vi "PH_DataViewer.panel.vi"(0 "object ref":refnum<vi>, 5 "error in (no error)":errorcluster) -> (19 "error out":errorcluster)   [LabVIEW 2014, in "PH_DataViewer.lvlib"]
doc: "By this VI a hardware switch can be monitored and switched. \n\nThe indicators \"FALSE\", \"TRUE\" and \"SWITCH STATE\" show the value of the Beckhoff-Tag: blue indicates bad tag status reference problems, darkgreen false and lightgreen true. If everything is working fine, \"FALSE\" and \"SWITCH STATE\" should show the same value, while \"TRUE\" has the opposite value. The caption of the sensors for \"FALSE\" and \"TRUE\" are taken out of the database. In case of only one or no sensor these GUI elements are not shown at all.\n\nThe oval button switches. It should be in the same state as the \"SWITCH STATE\" indicator. \n\n\"Delete Instance\" disconnects and removes the instance from the PCS.\n\n\nLicense Agreement for this software:\n\nCopyright (C)\nGesellschaft für Schwerionenforschung, GSI\nPlanckstr. 1\n64291 Darmstadt\nGermany\n\nContact: D.Beck@gsi.de \n\nThis program is free software; you can redistribute it and/or modify it under the terms of the GNU General Public License as published by the Free Software Foundation; either version 2 of the license, or (at your option) any later version.\n\nThis program is distributed in the hope that it will be useful, but WITHOUT ANYW ARRANTY; without even the implied warranty of MERCHANTABILITY or FITNESS FOR A PARTICULAR PURPOSE. See the GNU General License for more details (http://www.gnu.org).\n\nGesellschaft für Schwerionenforschung, GSI\nPlanckstr. 1, 64291 Darmstadt, Germany\nFor all questions and ideas contact: M.Richter@gsi.de, H.Brand@gsi.de or D.Beck@gsi.de.\nLast update: 18-DEC-2002"
uses:
  PH_DataViewer.lvlib
  PH_Calorimeter_USB/PH_Calorimeter_USB.Channel.ctl
  PH_Calorimeter_USB/PH_Calorimeter_USB.Channel Gain.ctl
  PH_gentec_Powermeter.Data.ctl
  PH_DataViewer.Device State.ctl
  PH_Common.PP PU Data.ctl
  PH_Basics/PH_StatusHandler/PH_StatusHandler.Status.ctl
  PH_PP_Trigger.Data.ctl
  PH_VacuumControl.Data.ctl
  PH_Blackbox.Data.ctl
  PH_PA_Chiller.Data.ctl
  PH_IEEE1394Camera.Data.ctl
  PH_IEEE1394Camera.Settings.ctl
  PH_ImageOperator.Data.ctl
  PH_Vision/PH_ImageCalibrator/PH_ImageCalibrator.Calibration Data - Version 1.ctl
  PH_Vision/PH_ImageOperator/PH_ImageOperator.Beam Analysis Data.ctl
  BNC555.Data.ctl
  PH_Common.PP PU Data Vers2.ctl
  PH_Sequencer.Data.ctl
  PH_BackreflectionMeas.Data.ctl
  PH_OceanOpticsSpectrometer.Data.ctl
  CS_Core/CSObj/CSObj.lvlib
  PH_Basics/PH_Common/PH_Common.lvlib
  PHELIX/PH_BackreflectionMeas/PH_BackreflectionMeas.lvlib
  PH_Devices/PH_OceanOpticsSpectrometer/PH_OceanOpticsSpectrometer.lvlib
  PH_Calorimeter_USB/PH_Calorimeter_USB.lvlib
  PH_Vision/PH_ImageOperator/PH_ImageOperator.lvlib
  PH_Basics/PH_StatusHandler/PH_StatusHandler.lvlib
  PH_Vision/PH_ImageCalibrator/PH_ImageCalibrator.lvlib
panel:
  out "OO Spectrometer":T1[](array[typedef])
  out "Backreflection Meas":T2[](array[typedef]) {"Waveform Data"."Initial X" format="%.2e"}
  in  "PP PU Data Version 2":T3={"Instance"="N/A", "Snapshot: Date"="N/A", "Snapshot: Time"="N/A", "PU in use?"=FALSE, "Time betweeen Shots [Min]"=0.0, "Waiting Time over?"=FALSE, "Voltage [V]"=0.0, "State"=0, "Timeout SM"=""} {"State" items=["no info", "off/false/out", "on/true/in", "Failure", "Alarm", "Status 1", "Status 2", "Status 3"]}
  out "f 2":dbl caption="mm"
  out "M":dbl
  out "Img Operators":T5[](array[typedef]) {"Energy"."State" items=["no info", "off/false", "on/true", "Failure", "Alarm"]; "Cam Settings"."Serial Number" format="%#_12g"; "Calibration"."Calibration data - Version 1"."Cam Settings"."Serial Number" format="%#_12g"; "Calibration"."Status" items=["no info", "off/false", "on/true", "Failure", "Alarm"]}
  out "Cams":T9[](array[typedef]) {"Cam Settings"."Serial Number" format="%#_12g"}
  out "PP PUs":T11[](array[typedef]) {"State" items=["no info", "off/false/out", "on/true/in", "Failure", "Alarm", "Status 1", "Status 2", "Status 3"]}
  out "Powermeters":T12[](array[typedef]) {"Device State" items=["no info", "off/false", "on/true", "Failure", "Alarm"]}
  in  "Empty":waveform(dbl)[](array[waveform])
  out "Current Meas Data":waveform(dbl)[][](array[waveform])
  in  "Main Tab":T13(tab)
  out "Sequencer Data":T14={"Instance"="N/A", "Snapshot: Date"="N/A", "Snapshot: Time"="N/A", "Shot Comment"=""}
  in  "Tab Opt Diagn":T15(tab)
  out "Time Calo":string
  out "Date Calo":string
  out "Graph":cluster{"Raw Data":dbl[], "Raw Data":dbl[]}(graph)
  out "Energy [J]":dbl format="%.3f"
  out "PH Calorimeter Device Config":T18 {"Channel Gain" items=["Range: +/- 10 V", "Range: +/- 2.5 V ", "Range: +/- 1 V", "Range: +/- 0.25 V", "Range: +/- 0.1 V", "Range: +/- 0.025 V"]; "Channel" items=["Channel 1", "Channel 2", "Channel 3", "Channel 4", "Channel 5", "Channel 6", "Channel 7", "Channel 8", "Channel 9", "Channel 10", "Channel 11", "Channel 12", "Channel 13", "Channel 14", "Channel 15", "Channel 16"]}
  out "Status Powermeter":u32(colorbox) caption="Powermeter"
  in  "Powermeter":u16(ring)
  out "Unit":string
  out "Current Value":dbl format="%#_3f"
  out "Serial Number":string
  out "Scaling Factor":dbl format="%#.3f"
  out "Trigger Level":dbl format="%#.3f"
  out "Time Powermeter":string
  out "Date Powermeter":string
  in  "Export Img Data":bool caption="Export Data"
  out "Cam Trigger":T19 caption="Trigger"
  out "Cam Settings":T20 caption="Settings" {"Serial Number" format="%#_15g"}
  in  "Cameras":u16(ring)
  out "Time Cams":string
  out "Date Cams":string
  out "Cam Image":T21(plugin-control) caption="Image"
  in  "Tab Img Op":T22(tab)
  in  "Export Op Img":bool caption="Export Data"
  out "Bg subtracted":bool
  out "Op Image":T21(plugin-control) caption="Image"
  out "f rel to major?":bool
  out "Energy":dbl caption="PiS" format="%#_8g"
  out "exp Energy":dbl caption="mJ"
  out "Energy on":bool caption="Energy"
  out "Analysis Type":u16(ring) items=["over all", "ROI"]
  out "BA: Factor for ROI":i32=3 caption="Factor"
  out "BA: Steps":i32=3 caption="Steps"
  out "CoG - Y":dbl caption="Pix"
  out "CoG - X":dbl caption="Pix"
  out "e":dbl caption="PixSum"
  out "f":dbl caption="°"
  out "Min Diam":dbl caption="Pix"
  out "Maj Diam":dbl caption="Pix"
  out "Beam Analysis":bool caption="Analysis"
  out "Position Type":u16(ring) items=["Nearfield", "Farfield"]
  out "D":dbl caption="mm"
  out "q":dbl caption="mrad"
  out "exp - Y":i32 caption="Pix"
  out "exp - X":i32 caption="Pix"
  out "Position":bool
  out "Min 1 %":dbl caption="Pix"
  out "Maj 1 %":dbl caption="Pix"
  out "Fit Gauss":bool
  out "Min Fit Order":i32
  out "Maj Fit Order":i32
  out "Min FWHM":dbl caption="Pix"
  out "Maj FWHM":dbl caption="Pix"
  in  "Export Min Trace":bool caption="Export Min"
  in  "Export Maj Trace":bool caption="Export Maj"
  out "Minor Trace":cluster{"Index":sgl[], dbl[]}[](graph)
  out "Major Trace":cluster{"Index":sgl[], dbl[]}[](graph)
  out "Cam Settings Operator":T20 caption="Settings" {"Serial Number" format="%#_15g"}
  out "Background Image":T21(plugin-control) caption="Image"
  in  "Export BG Img":bool caption="Export BG Image"
  out "Status Cali Data":T6 caption="Status" items=["no info", "off/false", "on/true", "Failure", "Alarm"]
  out "Calibration data":T23 {"Cam Settings"."Serial Number" format="%#_12g"}
  in  "Operators":u16(ring)
  out "Time Operators":string
  out "Date Operators":string
  in  "Export Data BRM":bool caption="Export Data"
  out "BRM Graph":waveform(dbl)[](graph)
  in  "Backreflection Measurement":u16(ring)
  out "Time BRM":string
  out "Date BRM":string
  in  "OO Spectrometer Instancelist":u16(ring)
  out "Time OO Spectro":string
  out "Date OO Spectro":string
  in  "Export OO Spectro Data":bool caption="Export Data"
  out "OO Spectrum":cluster{"Wavelength Bins":sgl[], sgl[]}(graph)
  in  "Tab PP":enum32{"Current Meas", "Power Units", "Misc"}(tab)
  in  "Export Current Meas Data":bool caption="Export Data"
  in  "Power Unit CM":u16(ring)
  out "current meas data indicator":waveform(dbl)[](graph) caption="Measurement data"
  out "Time Current Meas":string
  out "Date Current Meas":string
  out "Waiting Time [Min]":dbl
  out "State after Shot":T4 caption="PPMA Sequencer State" items=["no info", "off/false/out", "on/true/in", "Failure", "Alarm", "Status 1", "Status 2", "Status 3"]
  out "Timeout SM":string
  out "in use after Shot":bool caption="still on?"
  out "Time PU after Shot":string
  out "Date PU after Shot":string
  out "State before Shot":T4 caption="PPMA Sequencer State" items=["no info", "off/false/out", "on/true/in", "Failure", "Alarm", "Status 1", "Status 2", "Status 3"]
  out "Delay [s]":dbl
  out "Voltage [V]":dbl
  out "Waiting Time over":bool
  out "in use before Shot":bool caption="in use"
  out "Time PU before Shot":string
  out "Date PU before Shot":string
  out "Gate Gen Chan":string
  in  "Power Unit":u16(ring)
  out "Mercury Monitor":T24={"Device"="N/A", "Snapshot: Date"="N/A", "Snapshot: Time"="N/A", "State On/Off"=0, "State Alarm"=0, "Concentration [mg/m³]"=0.0, "On since"="N/A"} {"Concentration [mg/m³]" format="%#_9g"; "State Alarm" items=["no info", "off/false", "on/true", "Failure", "Alarm"]; "State On/Off" items=["no info", "off/false", "on/true", "Failure", "Alarm"]}
  out "Triggers":T25[](array[typedef])
  in  "Tab Timing":enum32{"BNC 555s", "SRDG 535s"}(tab)
  out "BNC555s":T27(array[cluster]) {"BNC555 ConfigData"."Configuration"."System"."To Gate Polarity" items=["Low", "High"]; "BNC555 ConfigData"."Configuration"."System"."To Trigger Edge" items=["Rising", "Falling"]; "BNC555 ConfigData"."Configuration"."System"."To Trigger Threshold" min=0.2 max=12 step=0.01 format="%.2f"; "BNC555 ConfigData"."Configuration"."System"."To DCycle Off Count" min=1 max=50000 step=1; "BNC555 ConfigData"."Configuration"."System"."To DCycle On Count" min=1 max=50000 step=1; "BNC555 ConfigData"."Configuration"."System"."To Burst Count" min=1 max=50000 step=1; "BNC555 ConfigData"."Configuration"."System"."To Trigger Mode" items=["Disabled", "Trigger", "Gate"]; "BNC555 ConfigData"."Configuration"."System"."To Mode" items=["Normal", "Single", "Burst", "DCycle"]; "BNC555 ConfigData"."Configuration"."System"."To Period" min=1e-06 max=20.0 step=1e-07 format="%.7f"; "BNC555 ConfigData"."Configuration"."System"."To State" items=["Disabled", "Enable"]; "BNC555 ConfigData"."Channel Array"."Channel Setup"."Ch Divide By Count" min=1 max=50000 step=1; "BNC555 ConfigData"."Channel Array"."Channel Setup"."Ch Burst Count" min=1 max=50000 step=1; "BNC555 ConfigData"."Channel Array"."Channel Setup"."Ch Mode" items=["Normal", "Single", "Burst", "Divide by"]; "BNC555 ConfigData"."Channel Array"."Channel Setup"."Ch Gate" items=["Disabled", "Enabled"]; "BNC555 ConfigData"."Channel Array"."Channel Setup"."Ch Gate Polarity" items=["Normal", "Complement"]; "BNC555 ConfigData"."Channel Array"."Channel Setup"."Ch Polarity" items=["Normal", "Complement"]; "BNC555 ConfigData"."Channel Array"."Channel Setup"."Ch Amplitude" min=1.99 max=12 step=0.01 format="%.2f"; "BNC555 ConfigData"."Channel Array"."Channel Setup"."Ch Output" items=["TTL", "Adjustable"]; "BNC555 ConfigData"."Channel Array"."Channel Setup"."Ch Delay" min=0.0 max=20.0 step=1e-09 format="%.9f"; "BNC555 ConfigData"."Channel Array"."Channel Setup"."Ch Width" min=4e-09 max=20.0 step=1e-09 format="%.9f"; "BNC555 ConfigData"."Channel Array"."Channel Setup"."Ch State" items=["Disabled", "Enable"]}
  out "SRDGs":T28(array[cluster]) {"Trigger Settings"."Burst Period" min=4 max=32766; "Trigger Settings"."Internal/Burst Rate (Hz)" min=0.001 max=1000000.0 format="%.3f"; "Trigger Settings"."external level (V)" min=-2.56 max=2.56 format="%.2f"; "Trigger Settings"."burst count" min=2 max=32766; "Trigger Settings"."trigger" scale=0.0..4.0; "Output Settings"."CH CD"."Mode" items=["TTL", "NIM", "ECL", "VAR"]; "Output Settings"."CH CD"."Offset (V)" min=-3.0 max=4.0 format="%.2f"; "Output Settings"."CH CD"."Amplitude (V)" min=-3.0 max=4.0 format="%.2f"; "Output Settings"."CH D"."Mode" items=["TTL", "NIM", "ECL", "VAR"]; "Output Settings"."CH D"."Offset (V)" min=-3.0 max=4.0 format="%.2f"; "Output Settings"."CH D"."Amplitude (V)" min=-3.0 max=4.0 format="%.2f"; "Output Settings"."CH C"."Mode" items=["TTL", "NIM", "ECL", "VAR"]; "Output Settings"."CH C"."Offset (V)" min=-3.0 max=4.0 format="%.2f"; "Output Settings"."CH C"."Amplitude (V)" min=-3.0 max=4.0 format="%.2f"; "Output Settings"."CH AB"."Mode" items=["TTL", "NIM", "ECL", "VAR"]; "Output Settings"."CH AB"."Offset (V)" min=-3.0 max=4.0 format="%.2f"; "Output Settings"."CH AB"."Amplitude (V)" min=-3.0 max=4.0 format="%.2f"; "Output Settings"."CH B"."Mode" items=["TTL", "NIM", "ECL", "VAR"]; "Output Settings"."CH B"."Offset (V)" min=-3.0 max=4.0 format="%.2f"; "Output Settings"."CH B"."Amplitude (V)" min=-3.0 max=4.0 format="%.2f"; "Output Settings"."CH A"."Mode" items=["TTL", "NIM", "ECL", "VAR"]; "Output Settings"."CH A"."Offset (V)" min=-3.0 max=4.0 format="%.2f"; "Output Settings"."CH A"."Amplitude (V)" min=-3.0 max=4.0 format="%.2f"; "Output Settings"."CH T0"."Mode" items=["TTL", "NIM", "ECL", "VAR"]; "Output Settings"."CH T0"."Offset (V)" min=-3.0 max=4.0 format="%.2f"; "Output Settings"."CH T0"."Amplitude (V)" min=-3.0 max=4.0 format="%.2f"; "Delay Settings"."CH D"."Delay (s)" format="%#_13g"; "Delay Settings"."CH D"."rel to" scale=0.0..3.0; "Delay Settings"."CH C"."Delay (s)" format="%#_13g"; "Delay Settings"."CH C"."rel to" scale=0.0..3.0; "Delay Settings"."CH B"."Delay (s)" format="%#_13g"; "Delay Settings"."CH B"."rel to" scale=0.0..3.0; "Delay Settings"."CH A"."Delay (s)" format="%#_13g"; "Delay Settings"."CH A"."rel to" scale=0.0..3.0}
  out "Chillers":T29[](array[typedef]) {"State Niveau" items=["no info", "off/false", "on/true", "Failure", "Alarm"]; "State Temperature" items=["no info", "off/false", "on/true", "Failure", "Alarm"]; "State Conductivity" items=["no info", "off/false", "on/true", "Failure", "Alarm"]; "State Flow" items=["no info", "off/false", "on/true", "Failure", "Alarm"]}
  out "Vac Controls":T30[](array[typedef])
  out "Black Boxes":T31[](array[typedef]) {"Status" items=["no info", "off/false", "on/true", "Failure", "Alarm", "Status 1", "Status 2", "Status 3"]}
  out "Path/File":path
  in  "Read Data":bool
  in  "Delete":bool
  out "loop counter":i32
  # "PCS"
  # "3.40"
  # "before Shot"
  # "after Shot"
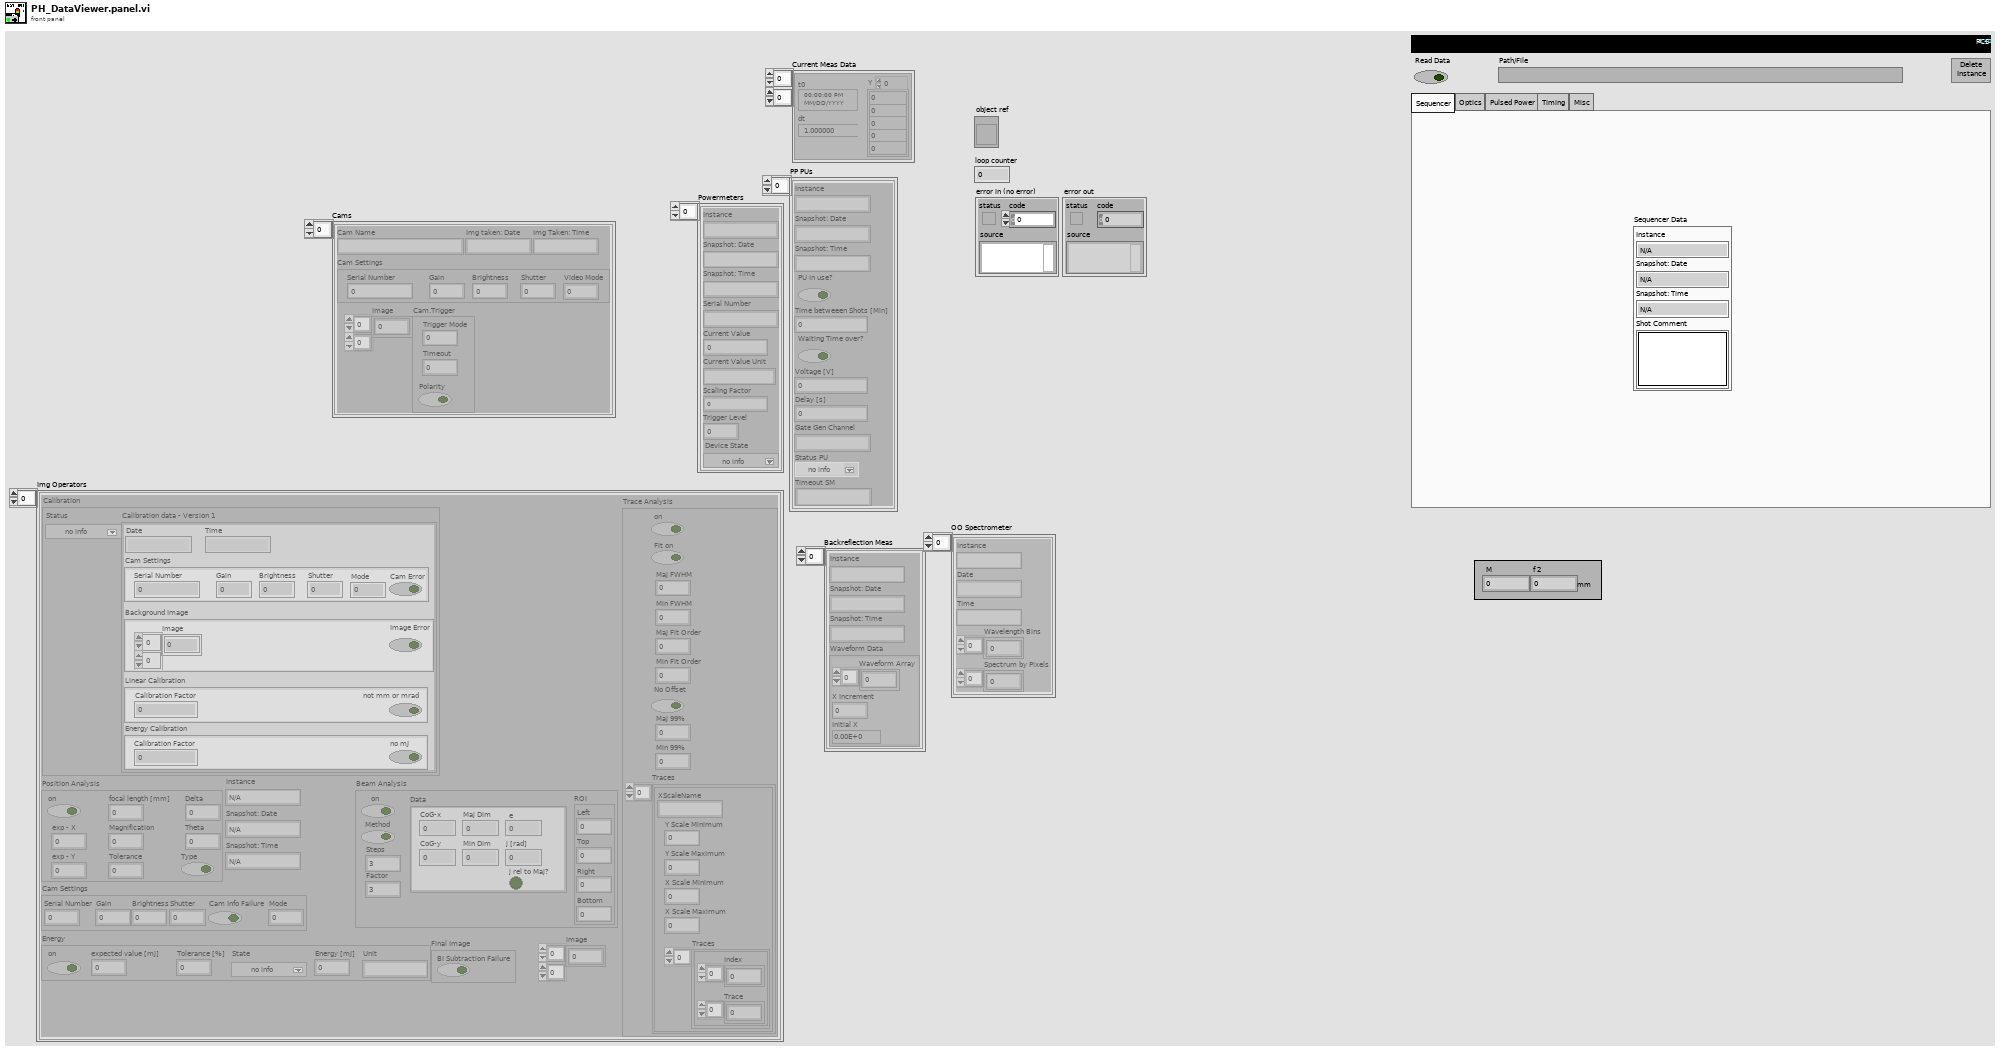
[diagram p1: front panel]
types:
  T1 = typedef "PH_DataViewer.lvlib/PH_OceanOpticsSpectrometer.Data.ctl" = cluster{"Instance":string, "Date":string, "Time":string, "Wavelength Bins":dbl[], "Spectrum by Pixels":dbl[]}
  T2 = typedef "PH_DataViewer.lvlib/PH_BackreflectionMeas.Data.ctl" = cluster{"Instance":string, "Snapshot: Date":string, "Snapshot: Time":string, "Waveform Data":cluster{"Waveform Array":dbl[], "X Increment":dbl, "Initial X":dbl}}
  T3 = typedef "PH_DataViewer.lvlib/PH_Common.PP PU Data Vers2.ctl" = cluster{"Instance":string, "Snapshot: Date":string, "Snapshot: Time":string, "PU in use?":bool, "Time betweeen Shots [Min]":dbl, "Waiting Time over?":bool, "Voltage [V]":dbl, "State":T4, "Timeout SM":string}
  T4 = typedef "PH_StatusHandler.lvlib/PH_StatusHandler.Status.ctl" = i16
  T5 = typedef "PH_DataViewer.lvlib/PH_ImageOperator.Data.ctl" = cluster{"Instance":string, "Snapshot: Date":string, "Snapshot: Time":string, "Calibration":cluster{"Status":T6, "Calibration data - Version 1":T7}, "Position Analysis":cluster{"on":bool, "exp - X":i32, "exp - Y":i32, "focal length [mm]":dbl, "Magnification":dbl, "Delta":dbl, "Theta":dbl, "Tolerance":dbl, "Type":bool}, "Beam Analysis":cluster{"on":bool, "Data":T8, "Method":bool, "Steps":i32, "Factor":i32, "ROI":cluster{"Left":i32, "Top":i32, "Right":i32, "Bottom":i32}}, "Cam Settings":cluster{"Serial Number":dbl, "Gain":i32, "Brightness":i32, "Shutter":i32, "Cam Info Failure":bool, "Mode":i32}, "Energy":cluster{"on":bool, "expected value [mJ]":dbl, "Tolerance [%]":dbl, "State":T6, "Energy [mJ]":dbl, "Unit":string}, "Image":dbl[][], "Final Image":cluster{"BI Subtraction Failure":bool}, "Trace Analysis":cluster{"on":bool, "Fit on":bool, "Maj FWHM":dbl, "Min FWHM":dbl, "Maj Fit Order":i32, "Min Fit Order":i32, "No Offset":bool, "Maj 99%":dbl, "Min 99%":dbl, "Traces":cluster{"XScaleName":string, "Y Scale Minimum":sgl, "Y Scale Maximum":sgl, "X Scale Minimum":sgl, "X Scale Maximum":sgl, "Traces":cluster{"Index":sgl[], "Trace":dbl[]}[]}[]}}
  T6 = typedef "PH_DataViewer.lvlib/PH_DataViewer.Device State.ctl" = i32
  T7 = typedef "PH_ImageCalibrator.lvlib/PH_ImageCalibrator.Calibration Data - Version 1.ctl" = cluster{"Date":string, "Time":string, "Cam Settings":cluster{"Serial Number":dbl, "Gain":i32, "Brightness":i32, "Shutter":i32, "Cam Error":bool, "Mode":i32}, "Background Image":cluster{"Image":dbl[][], "Image Error":bool}, "Linear Calibration":cluster{"Calibration Factor":dbl, "not mm or mrad":bool}, "Energy Calibration":cluster{"Calibration Factor":dbl, "no mJ":bool}}
  T8 = typedef "PH_ImageOperator.lvlib/PH_ImageOperator.Beam Analysis Data.ctl" = cluster{"CoG-x":sgl, "CoG-y":sgl, "Maj Dim":dbl, "Min Dim":dbl, "Ellipticity":dbl, "Azimuth Angle [rad]":dbl, "Azi Angle rel to Maj?":bool}
  T9 = typedef "PH_DataViewer.lvlib/PH_IEEE1394Camera.Data.ctl" = cluster{"Cam Name":string, "Img taken: Date":string, "Img Taken: Time":string, "Cam Settings":T10, "Image":sgl[][], "Cam.Trigger":cluster{"Trigger Mode":u16, "Timeout":u32, "Polarity":bool}}
  T10 = typedef "PH_DataViewer.lvlib/PH_IEEE1394Camera.Settings.ctl" = cluster{"Serial Number":dbl, "Gain":i32, "Brightness":i32, "Shutter":i32, "Video Mode":i32}
  T11 = typedef "PH_DataViewer.lvlib/PH_Common.PP PU Data.ctl" = cluster{"Instance":string, "Snapshot: Date":string, "Snapshot: Time":string, "PU in use?":bool, "Time betweeen Shots [Min]":dbl, "Waiting Time over?":bool, "Voltage [V]":dbl, "Delay [s]":dbl, "Gate Gen Channel":string, "State":T4, "Timeout SM":string}
  T12 = typedef "PH_DataViewer.lvlib/PH_gentec_Powermeter.Data.ctl" = cluster{"Instance":string, "Snapshot: Date":string, "Snapshot: Time":string, "Serial Number":string, "Current Value":dbl, "Current Value Unit":string, "Scaling Factor":dbl, "Trigger Level":dbl, "Device State":T6}
  T13 = enum32{"Sequencer", "Optics", "Pulsed Power", "Timing", "Misc"}
  T14 = typedef "PH_DataViewer.lvlib/PH_Sequencer.Data.ctl" = cluster{"Instance":string, "Snapshot: Date":string, "Snapshot: Time":string, "Shot Comment":string}
  T15 = enum32{"Calorimeter", "Powermeter", "Cams", "Operator", "Backreflection Meas", "OO Spectrometer"}
  T16 = typedef "PH_Calorimeter_USB.lvlib/PH_Calorimeter_USB.Channel.ctl" = u16
  T17 = typedef "PH_Calorimeter_USB.lvlib/PH_Calorimeter_USB.Channel Gain.ctl" = u16
  T18 = cluster{"Channel":T16, "Channel Gain":T17, "Device name":string, "Sensitivity [Vs/J]":dbl, "T 1/e [s]":dbl, "Serial No.":string}
  T19 = cluster{"Trigger Mode":u16, "Timeout":u32, "Polarity":bool}
  T20 = cluster{"Serial Number":dbl, "Gain":i32, "Brightness":i32, "Shutter":i32, "Mode":i32}
  T21 = typedef "IMAQ Image.ctl" = refnum<image>
  T22 = enum32{"Image", "Results", "Traces", "Cam Settings", "Bg Img", "Cali data"}
  T23 = cluster{"Date":string, "Time":string, "Cam Settings":cluster{"Serial Number":dbl, "Gain":i32, "Brightness":i32, "Shutter":i32, "Cam Error":bool, "Mode":i32}, "Background Image":cluster{"Image":dbl[][], "Image Error":bool}, "Linear Calibration":cluster{"Calibration Factor":dbl, "not mm nor mrad":bool}, "Energy Calibration":cluster{"Calibration Factor":dbl, "no mJ":bool}}
  T24 = cluster{"Device":string, "Snapshot: Date":string, "Snapshot: Time":string, "State On/Off":T6, "State Alarm":T6, "Concentration [mg/m³]":dbl, "On since":string}
  T25 = typedef "PH_DataViewer.lvlib/PH_PP_Trigger.Data.ctl" = cluster{"Instance":string, "Snapshot: Date":string, "Snapshot: Time":string, "last shot":string}
  T26 = typedef "PH_DataViewer.lvlib/BNC555.Data.ctl" = cluster{"Channel Array":cluster{"channel name (\"A\")":string, "Channel Setup":cluster{"Ch State":i8, "Ch Width":dbl, "Ch Delay":dbl, "Ch Output":i8, "Ch Amplitude":sgl, "Ch Polarity":i8, "Ch Gate Polarity":i8, "Ch Gate":i8, "Ch Mode":i8, "Ch Burst Count":i32, "Ch Divide By Count":i32}}[], "Configuration":cluster{"System":cluster{"To State":i8, "To Period":dbl, "To Mode":i8, "To Trigger Mode":i8, "To Burst Count":i32, "To DCycle On Count":i32, "To DCycle Off Count":i32, "To Trigger Threshold":sgl, "To Trigger Edge":i8, "To Gate Polarity":i8}}}
  T27 = cluster{"Object":string, "BNC555 ConfigData":T26}[]
  T28 = cluster{"Instance":string, "Snapshot: Date":string, "Snapshot: Time":string, "Delay Settings":cluster{"CH A":cluster{"rel to":u32, "Delay (s)":dbl}, "CH B":cluster{"rel to":u32, "Delay (s)":dbl}, "CH C":cluster{"rel to":u32, "Delay (s)":dbl}, "CH D":cluster{"rel to":u32, "Delay (s)":dbl}}, "Output Settings":cluster{"CH T0":cluster{"Inversion":bool, "Amplitude (V)":dbl, "Offset (V)":dbl, "Mode":i32, "Load":bool}, "CH A":cluster{"Inversion":bool, "Amplitude (V)":dbl, "Offset (V)":dbl, "Mode":i32, "Load":bool}, "CH B":cluster{"Inversion":bool, "Amplitude (V)":dbl, "Offset (V)":dbl, "Mode":i32, "Load":bool}, "CH AB":cluster{"Inversion":bool, "Amplitude (V)":dbl, "Offset (V)":dbl, "Mode":i32, "Load":bool}, "CH C":cluster{"Inversion":bool, "Amplitude (V)":dbl, "Offset (V)":dbl, "Mode":i32, "Load":bool}, "CH D":cluster{"Inversion":bool, "Amplitude (V)":dbl, "Offset (V)":dbl, "Mode":i32, "Load":bool}, "CH CD":cluster{"Inversion":bool, "Amplitude (V)":dbl, "Offset (V)":dbl, "Mode":i32, "Load":bool}}, "Trigger Settings":cluster{"trigger":u32, "Impedance":bool, "Slope":bool, "burst count":i32, "external level (V)":sgl, "Internal/Burst Rate (Hz)":dbl, "Burst Period":i32}}[]
  T29 = typedef "PH_DataViewer.lvlib/PH_PA_Chiller.Data.ctl" = cluster{"Instance":string, "Snapshot: Date":string, "Snapshot: Time":string, "State Flow":T6, "State Conductivity":T6, "State Temperature":T6, "State Niveau":T6}
  T30 = typedef "PH_DataViewer.lvlib/PH_VacuumControl.Data.ctl" = cluster{"Instance":string, "Snapshot: Date":string, "Snapshot: Time":string, "Channels":cluster{"Gauge":string, "Value (mbar)":dbl, "Limit (mbar)":dbl}[]}
  T31 = typedef "PH_DataViewer.lvlib/PH_Blackbox.Data.ctl" = cluster{"Instance":string, "Snapshot: Date":string, "Snapshot: Time":string, "Remote Controlled?":bool, "Status":i32}
  T32 = typedef "PH_DataViewer.lvlib/PH_DataViewer.i attribute.ctl" = cluster{"Images":cluster{"CAM":cluster{string, u32}, "BACKGROUND":cluster{string, u32}, "OPERATOR":cluster{string, u32}}, "Cam Operator GUI Refs":cluster{"Date Operators":refnum<vi>, "Time Operators":refnum<vi>, "Status Cali Data":refnum<vi>, "Calibration data":refnum<vi>, "Background Image":refnum<vi>, "Bg subtracted":refnum<vi>, "Op Image":refnum<vi>, "Cam Settings Operator":refnum<vi>, "Energy on":refnum<vi>, "exp Energy":refnum<vi>, "Energy":refnum<vi>, "Beam Analysis":refnum<vi>, "Analysis Type":refnum<vi>, "BA: Steps":refnum<vi>, "BA: Factor for ROI":refnum<vi>, "CoG - X":refnum<vi>, "CoG - Y":refnum<vi>, "Maj Diam":refnum<vi>, "Min Diam":refnum<vi>, "Phi":refnum<vi>, "Epsilon":refnum<vi>, "Phi rel to maj":refnum<vi>, "Position":refnum<vi>, "Position Type":refnum<vi>, "exp - X":refnum<vi>, "exp - Y":refnum<vi>, "Magni":refnum<vi>, "Foc Length":refnum<vi>, "Delta":refnum<vi>, "Theta":refnum<vi>, "Fit Gauss":refnum<vi>, "Maj Fit Order":refnum<vi>, "Min Fit Order":refnum<vi>, "Maj FWHM":refnum<vi>, "Min FWHM":refnum<vi>, "Maj 1 %":refnum<vi>, "Min 1 %":refnum<vi>}}
  T33 = typedef "PH_DataViewer.lvlib/PH_Calorimater_USB.Data.ctl" = cluster{"PH Calorimeter Device Config":T34, "Output Rate [Hz]":i32, "Offset time [s]":dbl, "Taken + Calc: Date":string, "Taken + Calc: Time":string, "Raw Data":dbl[][], "Energy [J]":dbl}
  T34 = typedef "PH_Calorimeter_USB.lvlib/PH_Calorimeter_USB.Device Config.ctl" = cluster{"Channel":T16, "Channel Gain":T17, "Device name":string, "Sensitivity":dbl, "T 1/e":dbl, "Serial No.":string}
  T35 = typedef "PH_DataViewer.lvlib/PH_CurrentMeas.Data.ctl" = cluster{"Instance":string, "Snapshot: Date":string, "Snapshot: Time":string, "PU Data":cluster{"Data":waveform(dbl)[], "PU Name":string}[]}
  T36 = typedef "PH_DataViewer.lvlib/PH_Mercury_Monitor.Data.ctl" = cluster{"Device":string, "Snapshot: Date":string, "Snapshot: Time":string, "State On/Off":T6, "State Alarm":T6, "Concentration [mg/m³]":dbl, "On since":string}
  T37 = cluster{"Black Boxes":T31[], "Calorimeters":T33[], "Current Meas'":T35[], "Powermeters":T12[], "Cams":T9[], "Img Operators":T5[], "Mercury Monitors":T36[], "Chillers":T29[], "Triggers":T25[], "Vac Controls":T30[], "PP PUs":T11[], "BNC555s":cluster{"Object":string, "BNC555 ConfigData":T26}[]}
  T38 = typedef "PH_DataViewer.lvlib/PHELIX_Data_Vers2.ctl" = cluster{"Black Boxes":T31[], "Calorimeters":T33[], "Current Meas'":T35[], "Powermeters":T12[], "Cams":T9[], "Img Operators":T5[], "Mercury Monitors":T36[], "Chillers":T29[], "Triggers":T25[], "Vac Controls":T30[], "PP PUs":T3[], "BNC555s":cluster{"Object":string, "BNC555 ConfigData":T26}[], "SRDG535s":T39[], "Sequencer Data":T14}
  T39 = typedef "PH_DataViewer.lvlib/SRDG535.Data.ctl" = cluster{"Instance":string, "Snapshot: Date":string, "Snapshot: Time":string, "Delay Settings":T40, "Output Settings":T41, "Trigger Settings":T43}
  T40 = typedef "SRDG535.lvlib/SRDG535.Delay.ctl" = cluster{"CH A":cluster{"rel to":u32, "Delay (s)":dbl}, "CH B":cluster{"rel to":u32, "Delay (s)":dbl}, "CH C":cluster{"rel to":u32, "Delay (s)":dbl}, "CH D":cluster{"rel to":u32, "Delay (s)":dbl}}
  T41 = typedef "SRDG535.lvlib/SRDG535.Output.ctl" = cluster{"CH T0":T42, "CH A":T42, "CH B":T42, "CH AB":T42, "CH C":T42, "CH D":T42, "CH CD":T42}
  T42 = typedef "SRDG535.lvlib/SRDG535.Channel Output.ctl" = cluster{"Inversion":bool, "Amplitude (V)":dbl, "Offset (V)":dbl, "Mode":i32, "Load":bool}
  T43 = typedef "SRDG535.lvlib/SRDG535.Trigger.ctl" = cluster{"trigger":u32, "Impedance":bool, "Slope":bool, "burst count":i32, "external level (V)":sgl, "Internal/Burst Rate (Hz)":dbl, "Burst Period":i32}
  T44 = typedef "PH_DataViewer.lvlib/PHELIX_Data_Vers3.ctl" = cluster{"Black Boxes":T31[], "Calorimeters":T33[], "Current Meas'":T35[], "Powermeters":T12[], "Cams":T9[], "Img Operators":T5[], "Mercury Monitors":T36[], "Chillers":T29[], "Triggers":T25[], "Vac Controls":T30[], "PP PUs":T3[], "BNC555s":cluster{"Object":string, "BNC555 ConfigData":T26}[], "SRDG535s":T39[], "Sequencer Data":T14, "Backreflection Meas":T2[]}
  T45 = typedef "PH_DataViewer.lvlib/PHELIX_Data_Vers4.ctl" = cluster{"Black Boxes":T31[], "Calorimeters":T33[], "Current Meas'":T35[], "Powermeters":T12[], "Cams":T9[], "Img Operators":T5[], "Mercury Monitors":T36[], "Chillers":T29[], "Triggers":T25[], "Vac Controls":T30[], "PP PUs":T3[], "BNC555s":cluster{"Object":string, "BNC555 ConfigData":T26}[], "SRDG535s":T39[], "Sequencer Data":T14, "Backreflection Meas":T2[], "OO Spectrometer":T1[]}
  T46 = cluster{"XScaleName":string, "Y Scale Minimum":sgl, "Y Scale Maximum":sgl, "X Scale Minimum":sgl, "X Scale Maximum":sgl, "Traces":cluster{"Index":sgl[], "Trace":dbl[]}[]}[]
  T47 = cluster{"XScaleName":string, "Y Scale Minimum":sgl, "Y Scale Maximum":sgl, "X Scale Minimum":sgl, "X Scale Maximum":sgl, "Traces":cluster{"Index":sgl[], "Trace":dbl[]}[]}
  T48 = cluster{"Wavelength Bins":dbl[], "Spectrum by Pixels":dbl[]}
  T49 = typedef "PH_IEEE1394Camera.Data.ctl" = cluster{"Cam Name":string, "Img taken: Date":string, "Img Taken: Time":string, "Cam Settings":T50, "Image":sgl[][], "Cam.Trigger":cluster{"Trigger Mode":u16, "Timeout":u32, "Polarity":bool}}
  T50 = typedef "PH_IEEE1394Camera.Settings.ctl" = cluster{"Serial Number":dbl, "Gain":i32, "Brightness":i32, "Shutter":i32, "Video Mode":i32}
  T51 = cluster{"Waveform Array":dbl[], "X Increment":dbl, "Initial X":dbl}
  T52 = typedef "PH_OceanOpticsSpectrometer.lvlib/PH_OceanOpticsSpectrometer.Data.ctl" = cluster{"Instance":string, "Date":string, "Time":string, "Wavelength Bins":dbl[], "Spectrum by Pixels":dbl[]}
  T53 = typedef "PH_gentec_Powermeter.Data.ctl" = cluster{"Instance":string, "Snapshot: Date":string, "Snapshot: Time":string, "Serial Number":string, "Current Value":dbl, "Current Value Unit":string, "Scaling Factor":dbl, "Trigger Level":dbl, "Device State":T54}
  T54 = typedef "Device State.ctl" = i32
  T55 = typedef "PH_Common.PP PU Data.ctl" = cluster{"Instance":string, "Snapshot: Date":string, "Snapshot: Time":string, "PU in use?":bool, "Time betweeen Shots [Min]":dbl, "Waiting Time over?":bool, "Voltage [V]":dbl, "Delay [s]":dbl, "Gate Gen Channel":string, "State":T56, "Timeout SM":string}
  T56 = typedef "Status.ctl" = i16
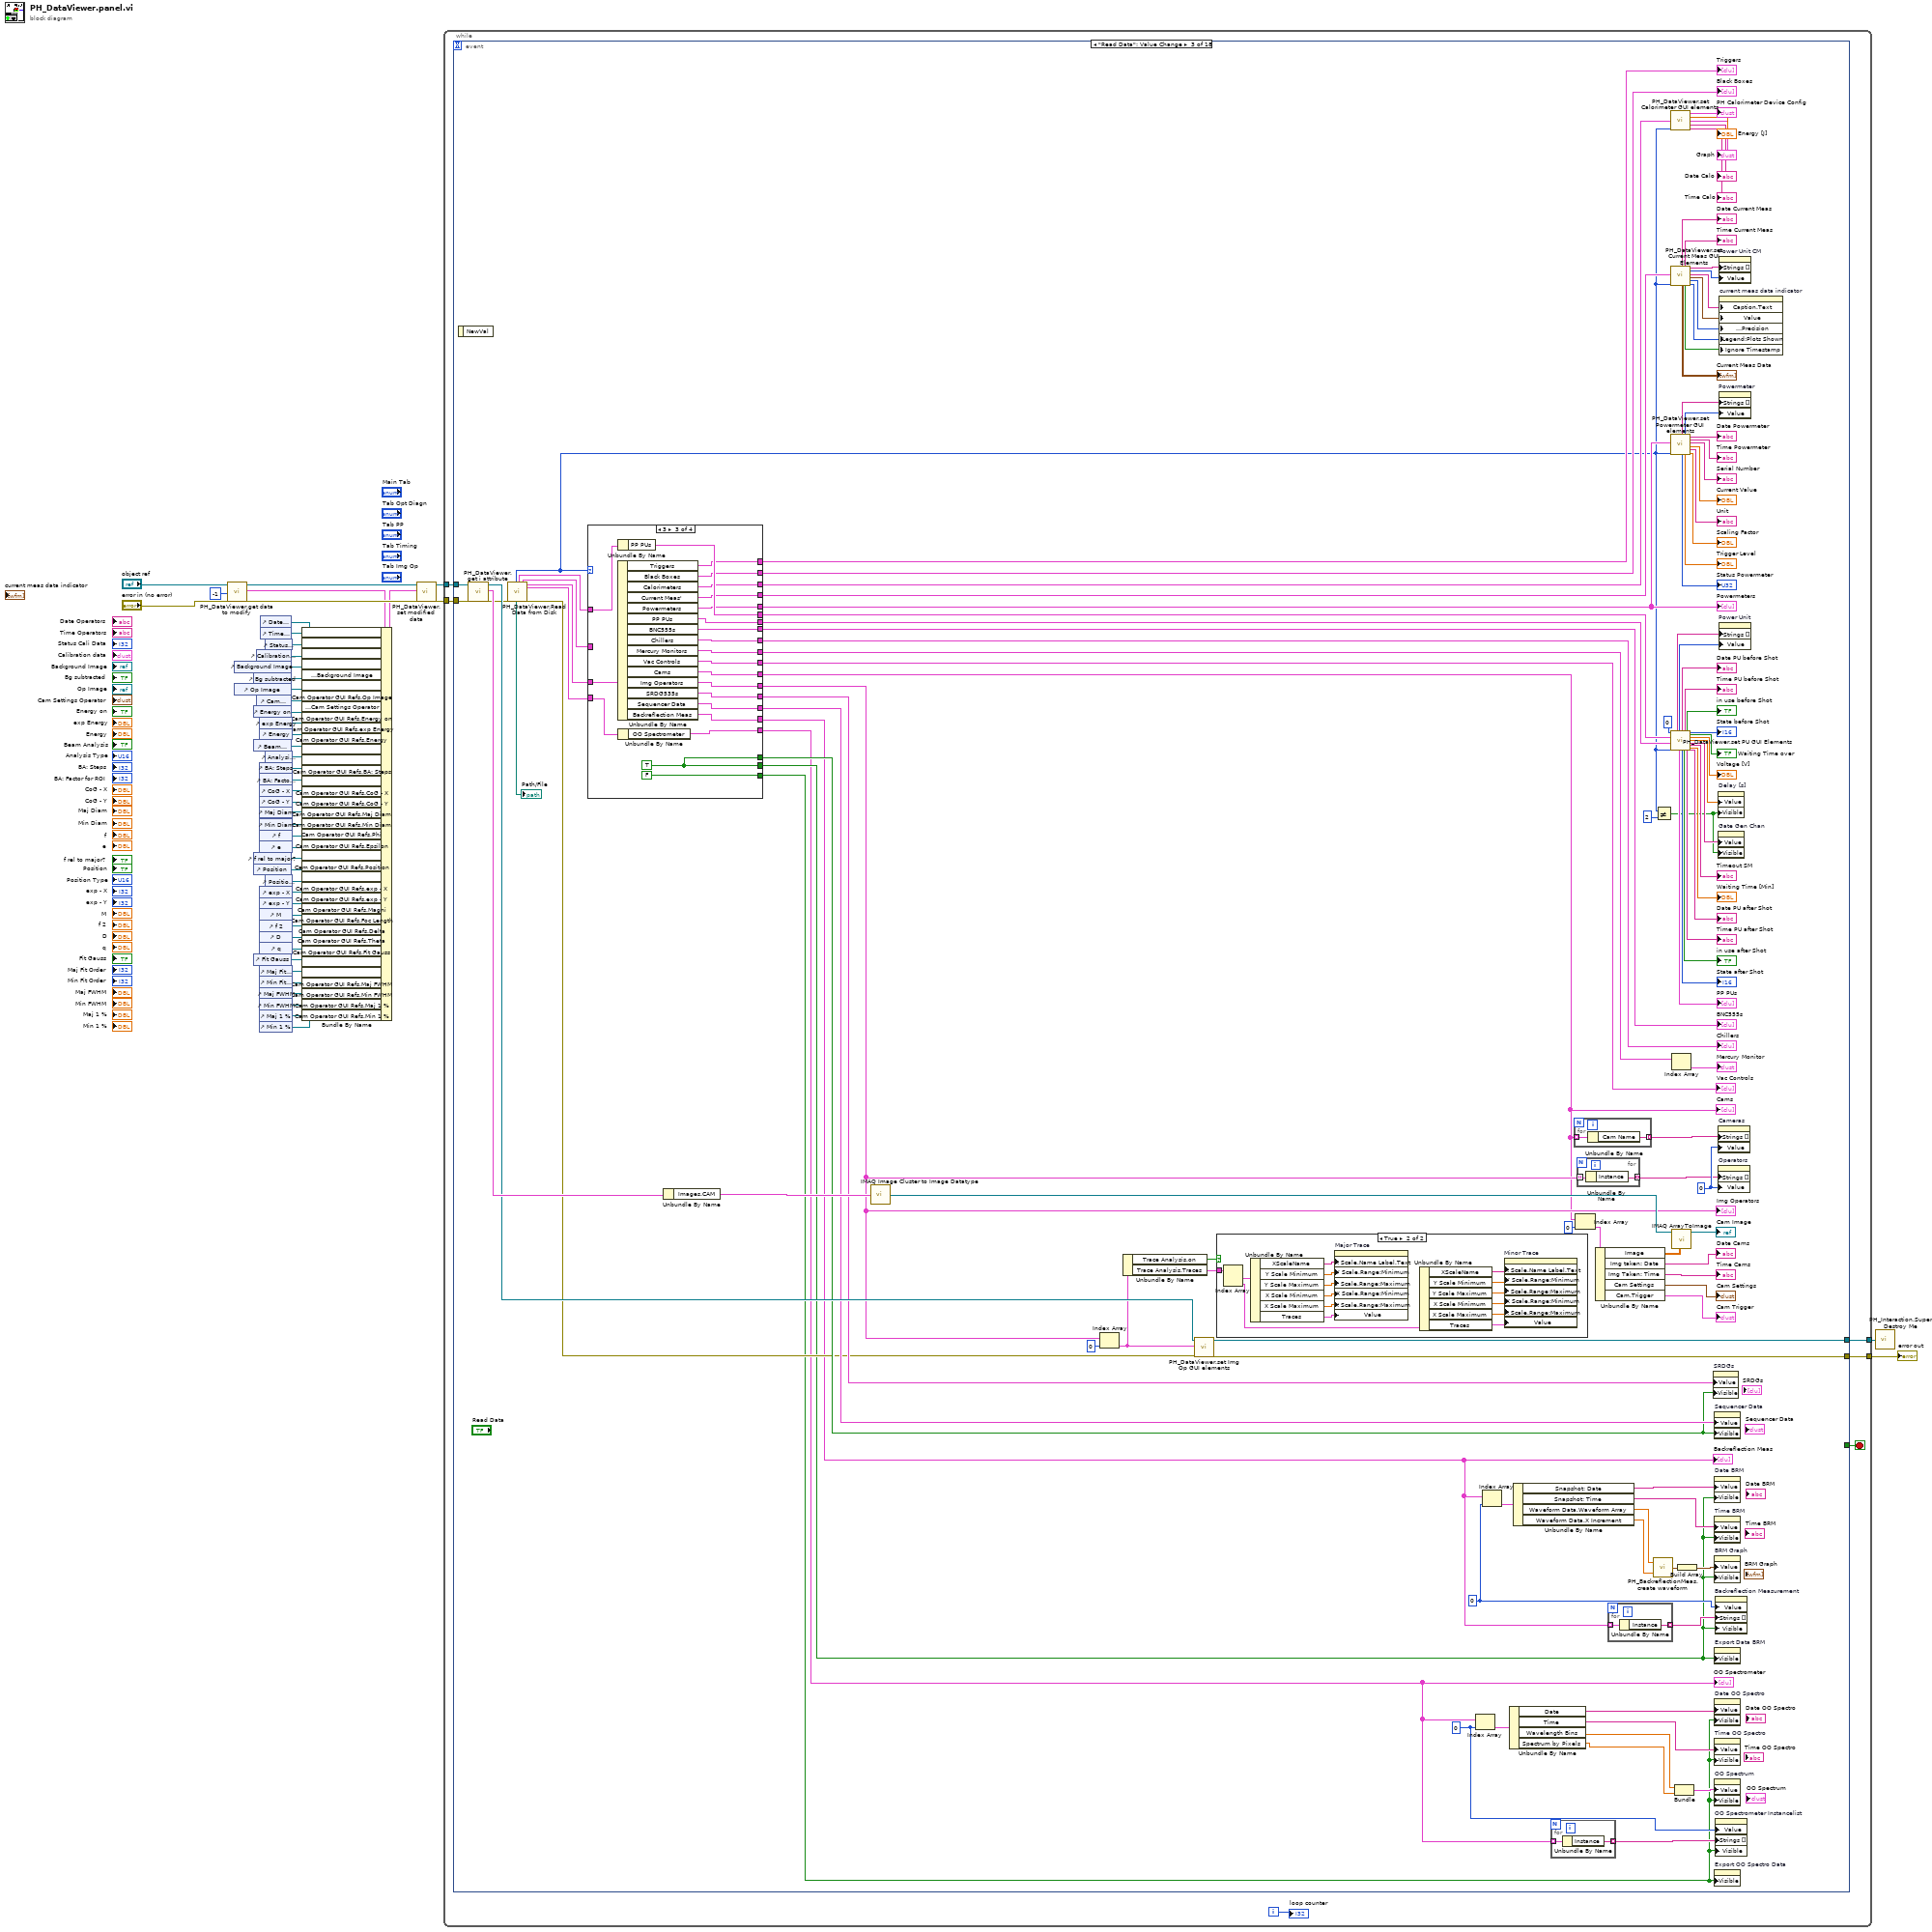
[diagram p0: block diagram]
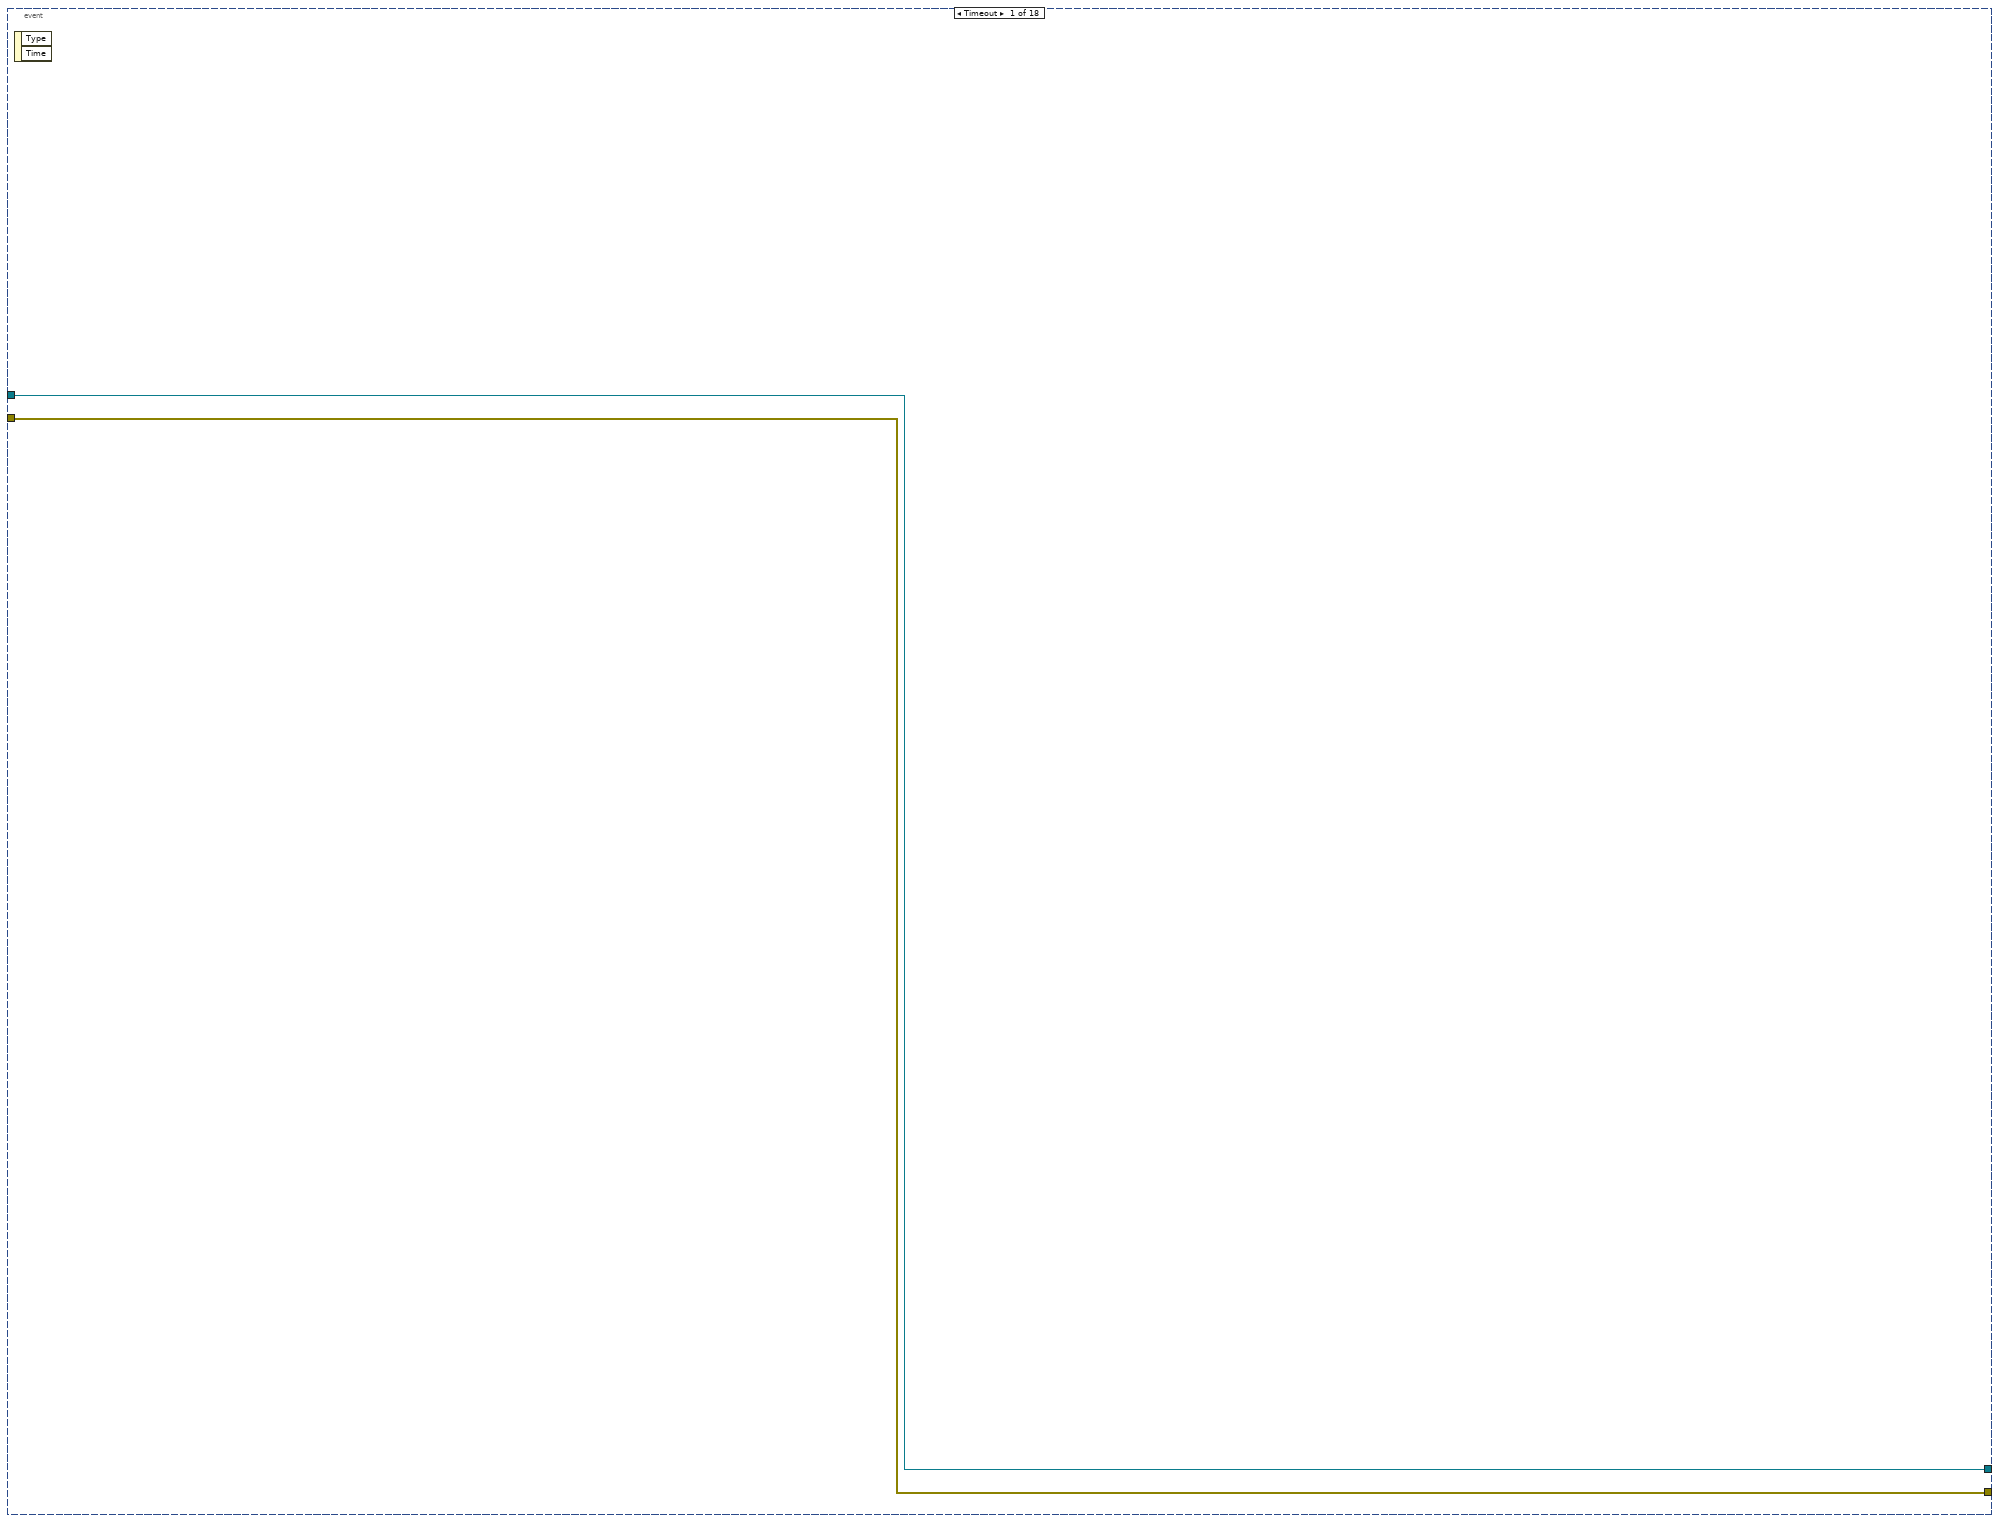
[diagram p2: hidden frame]
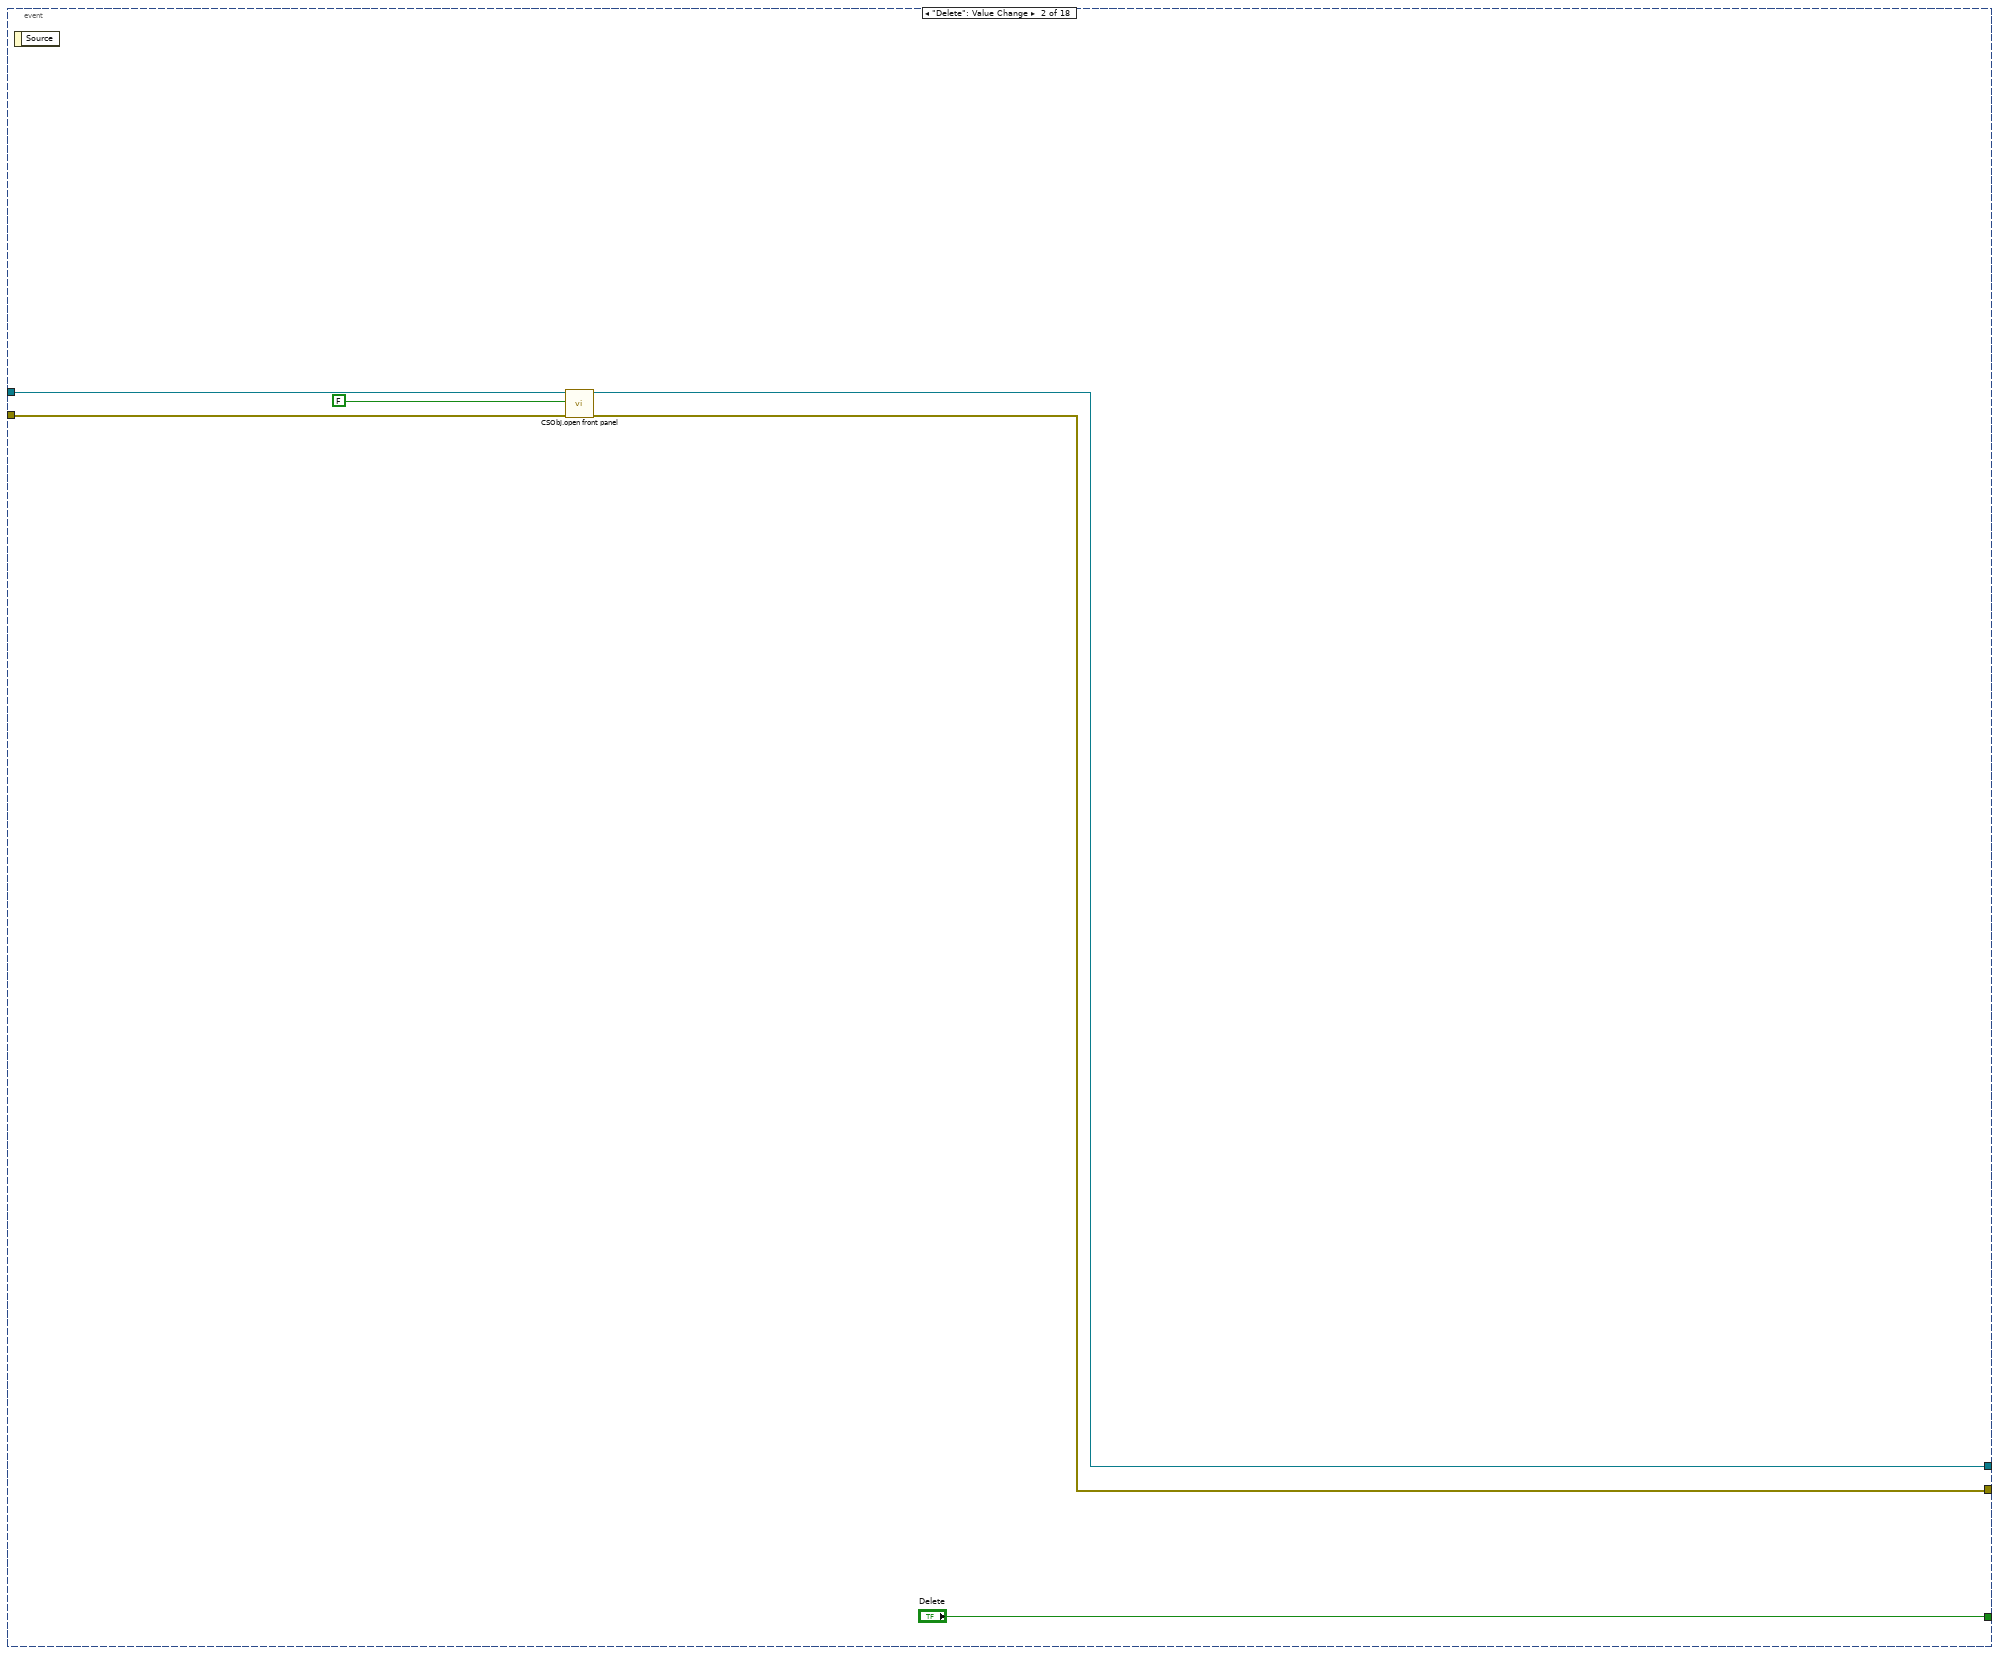
[diagram p3: hidden frame]
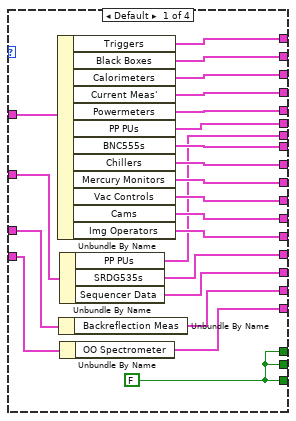
[diagram p4: hidden frame]
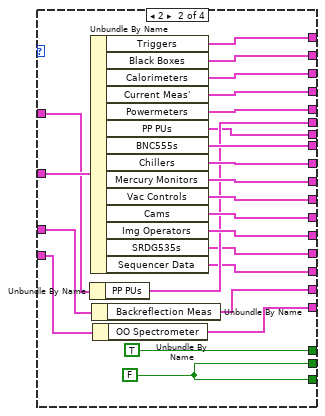
[diagram p5: hidden frame]
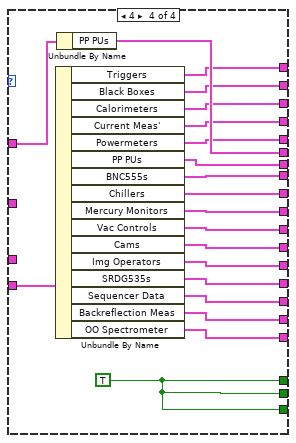
[diagram p6: hidden frame]
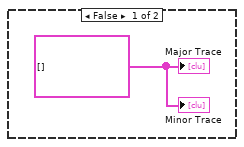
[diagram p7: hidden frame]
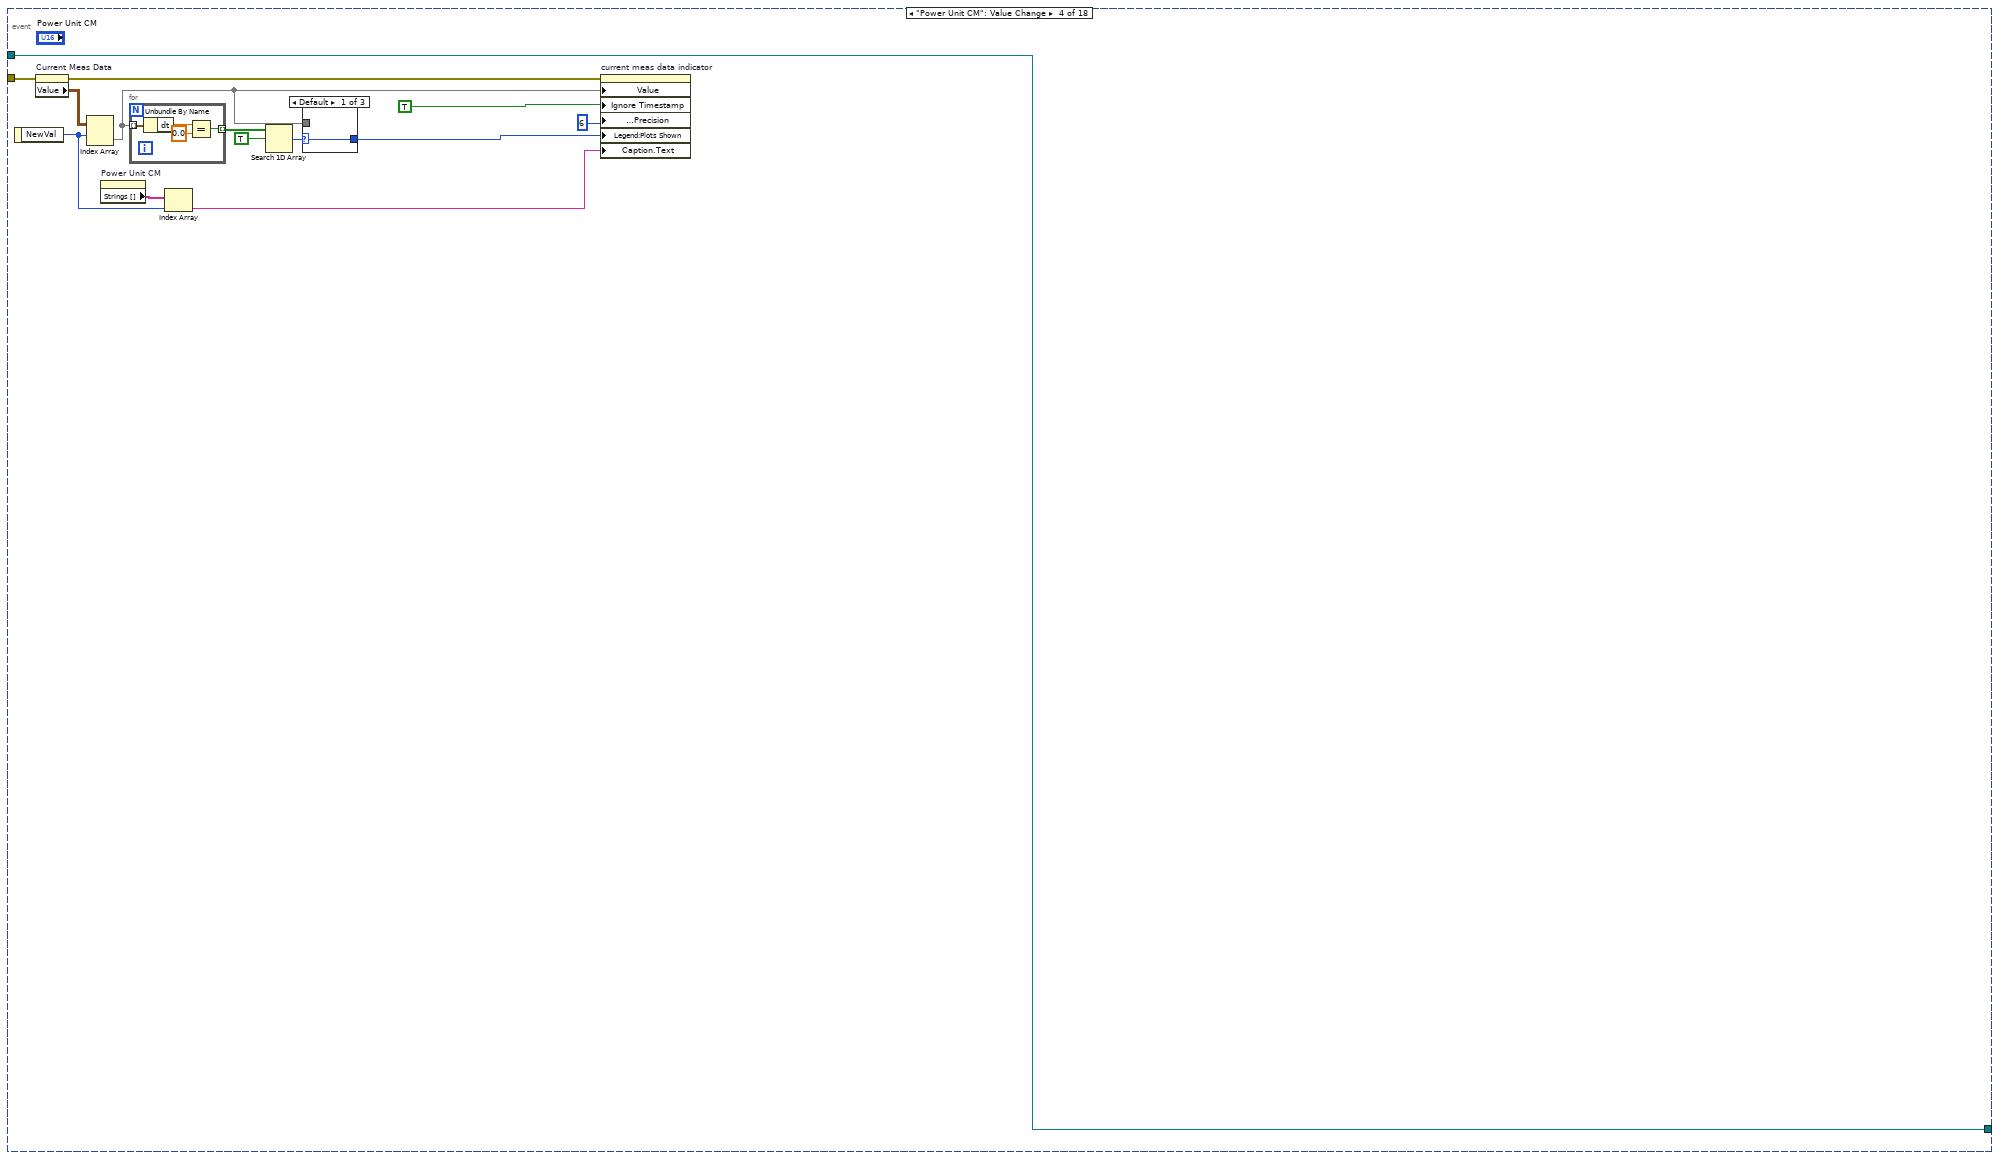
[diagram p8: hidden frame]
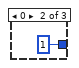
[diagram p9: hidden frame]
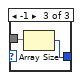
[diagram p10: hidden frame]
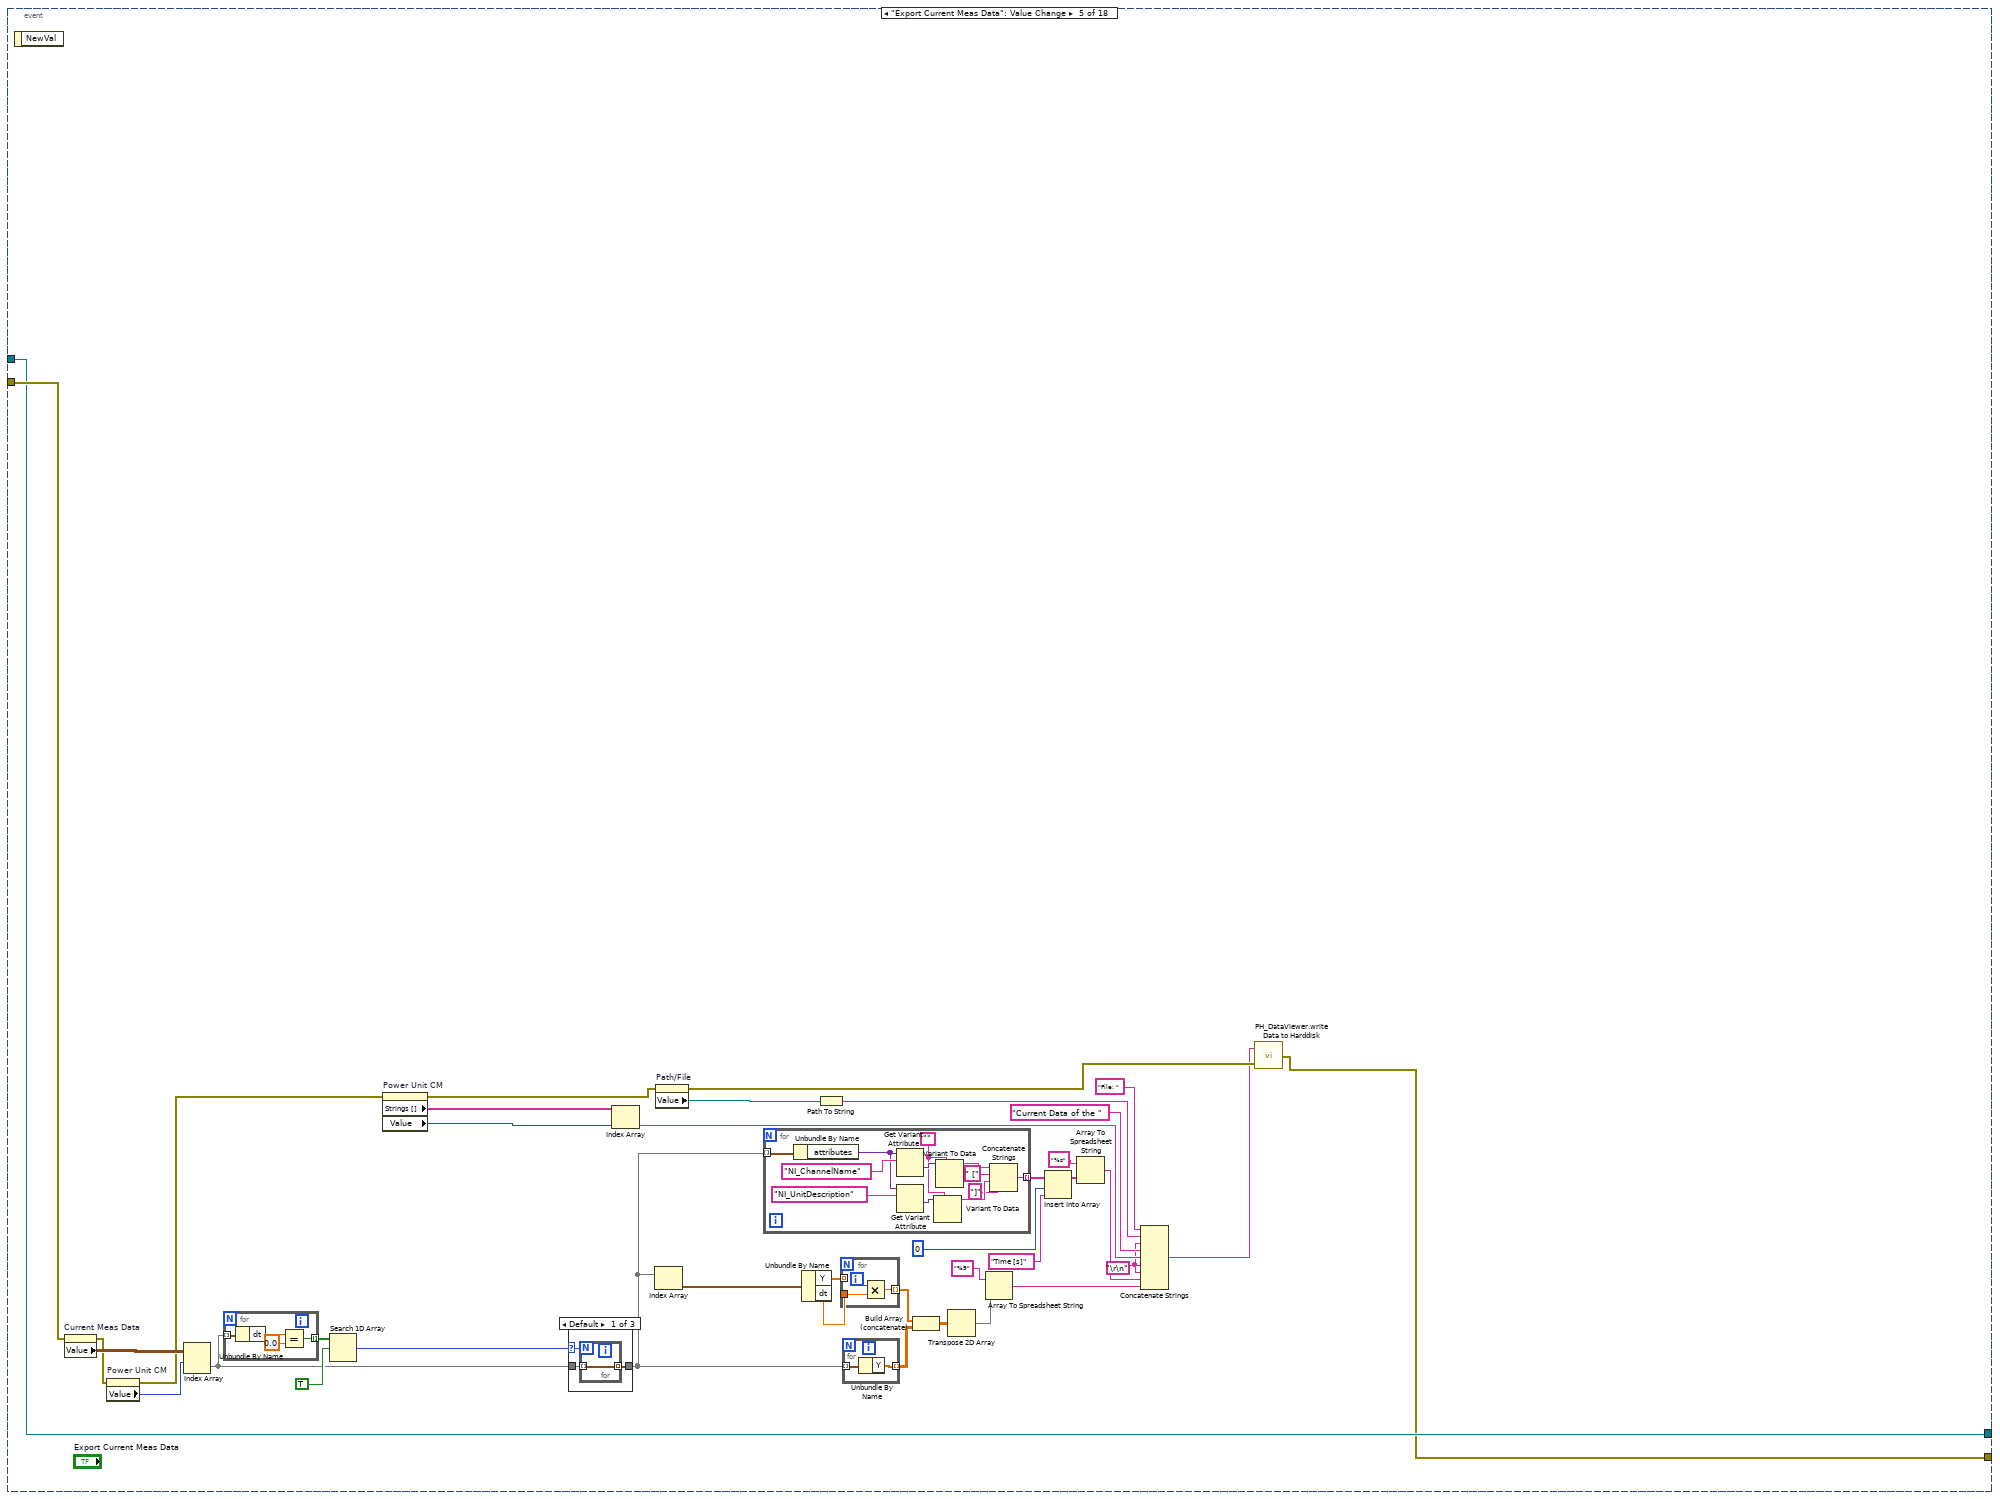
[diagram p11: hidden frame]
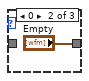
[diagram p12: hidden frame]
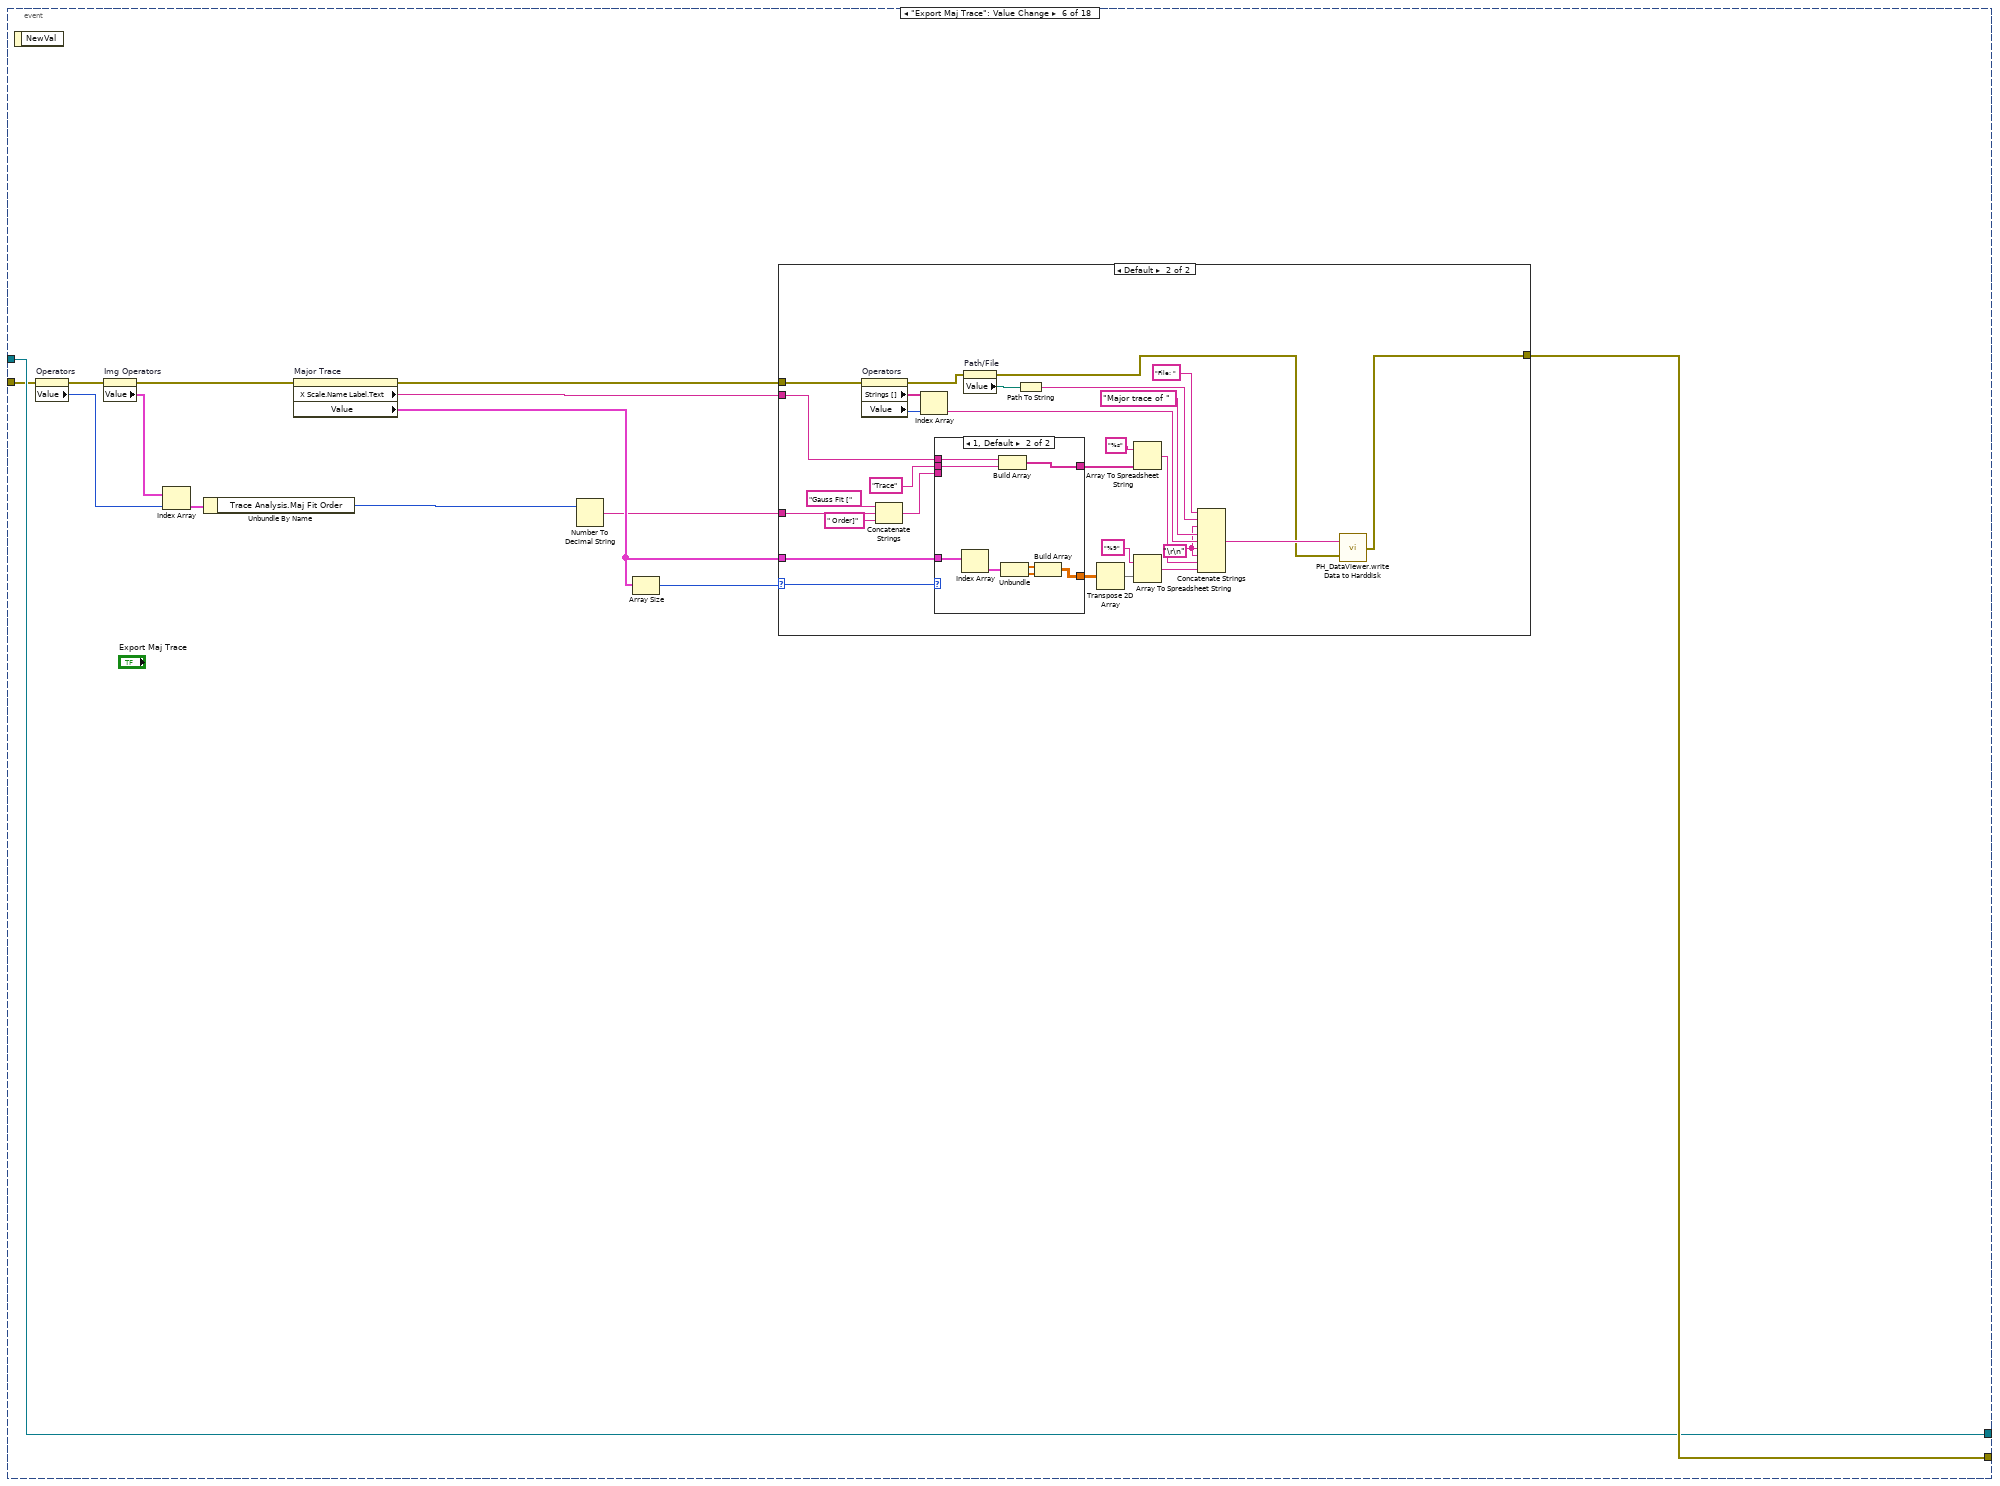
[diagram p14: hidden frame]
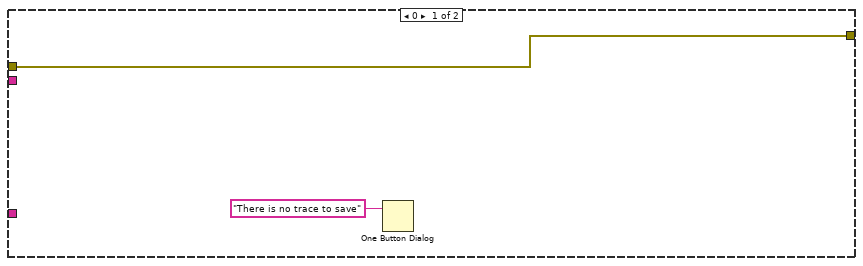
[diagram p15: hidden frame]
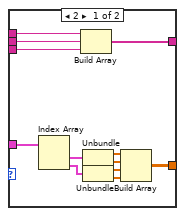
[diagram p16: hidden frame]
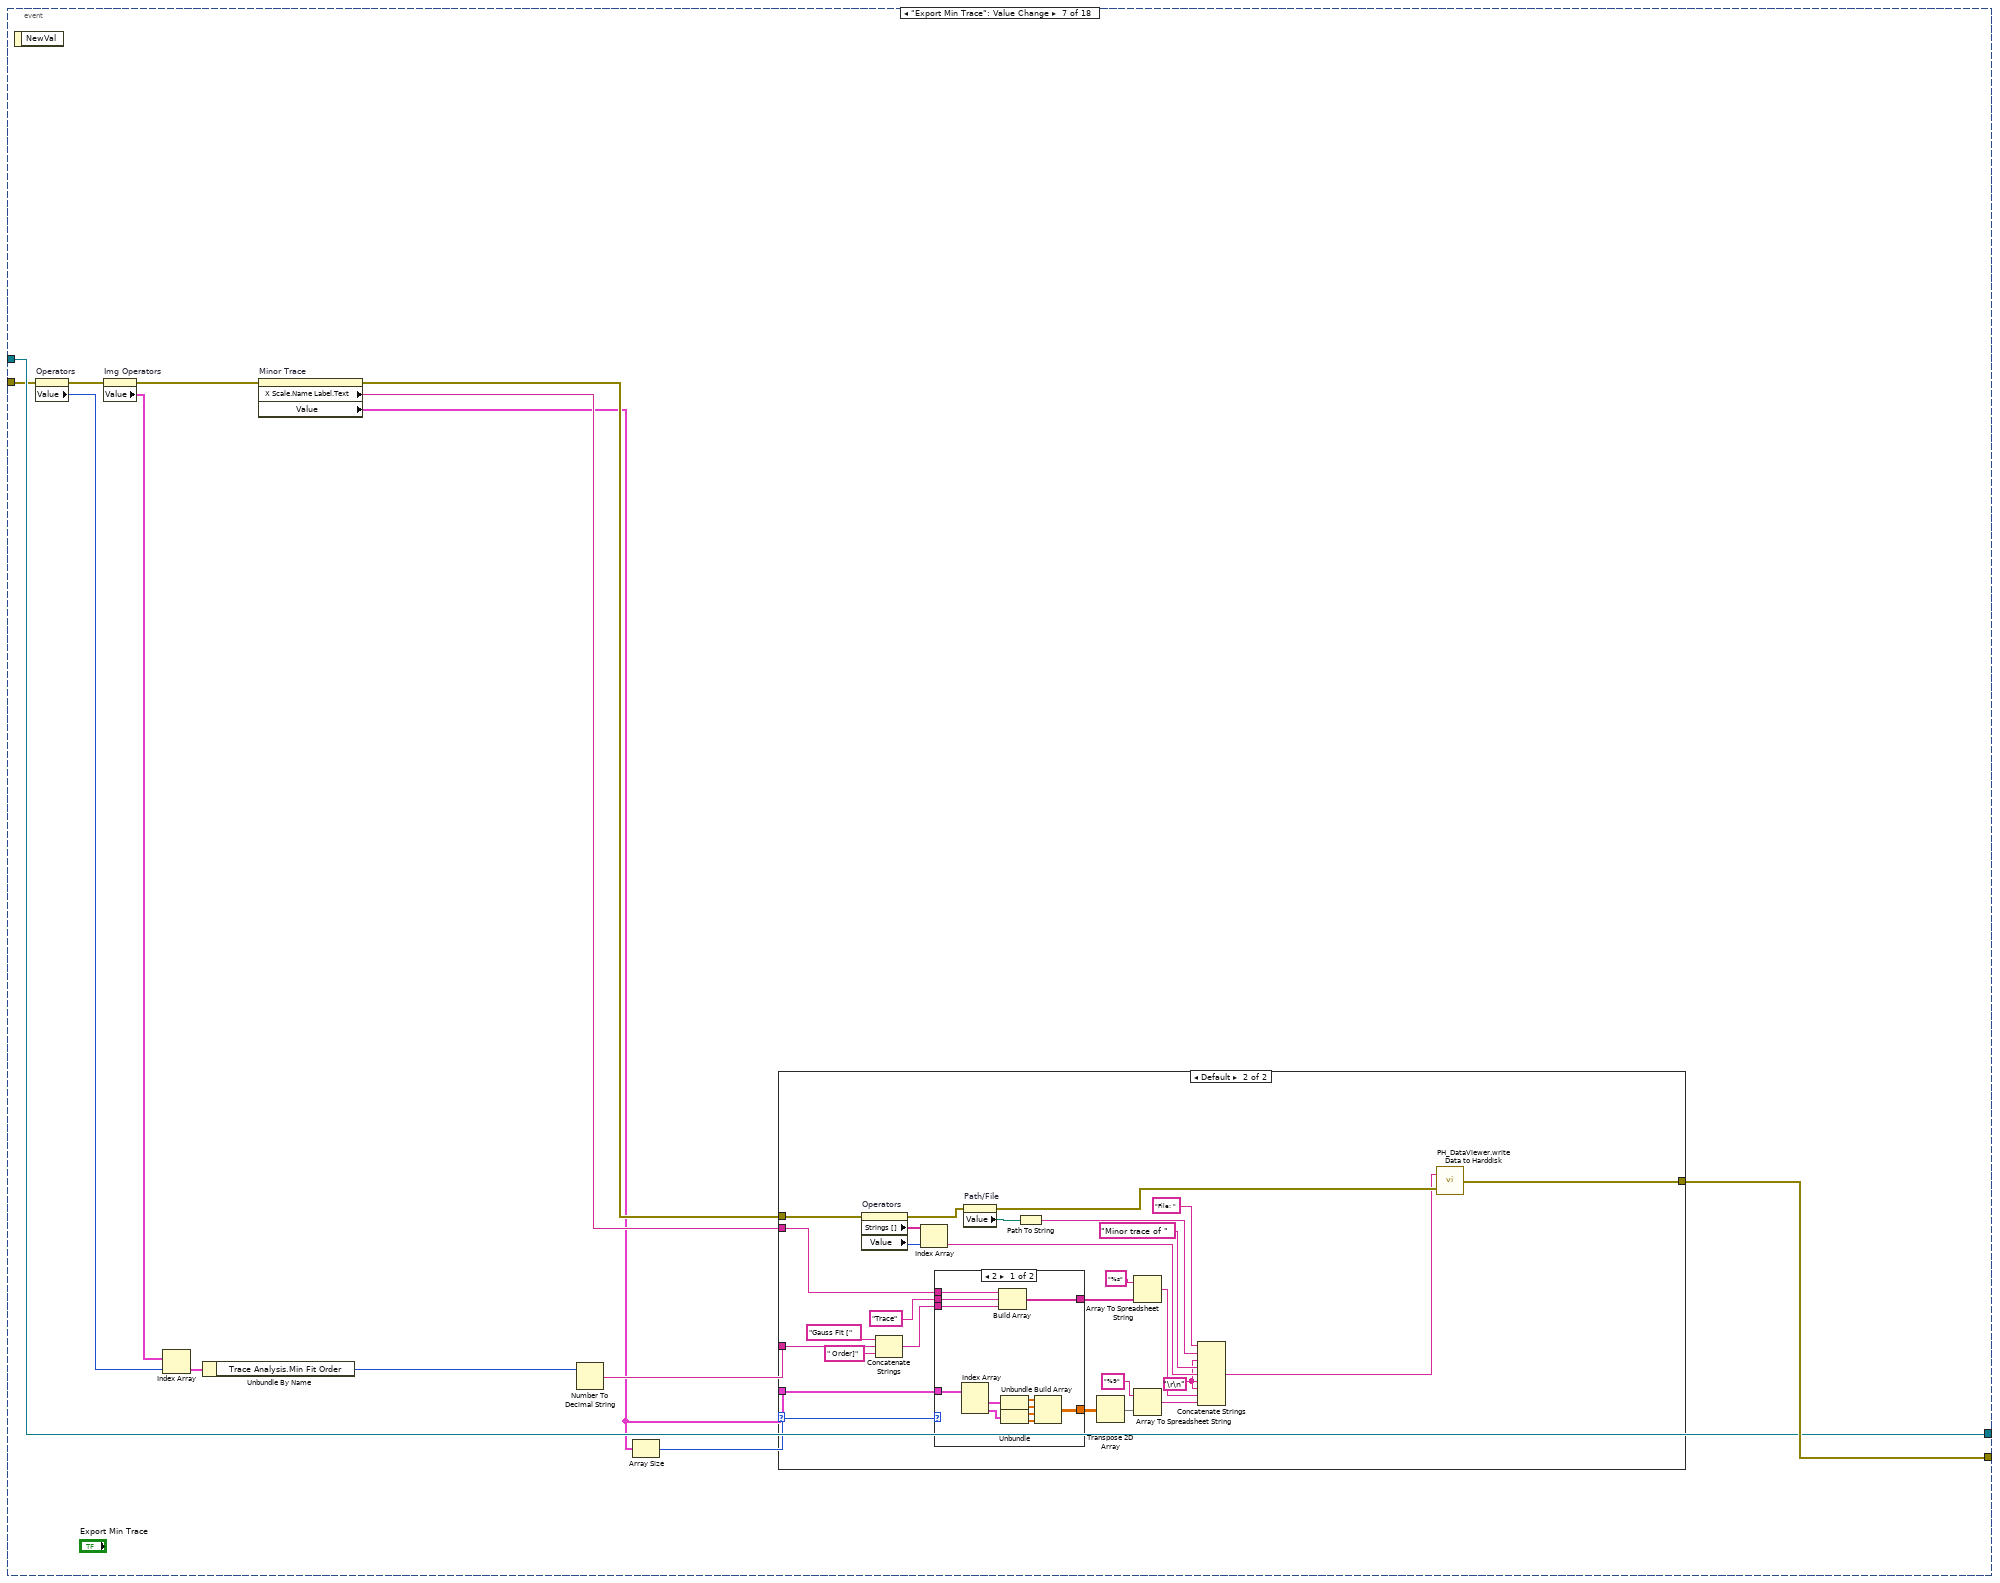
[diagram p17: hidden frame]
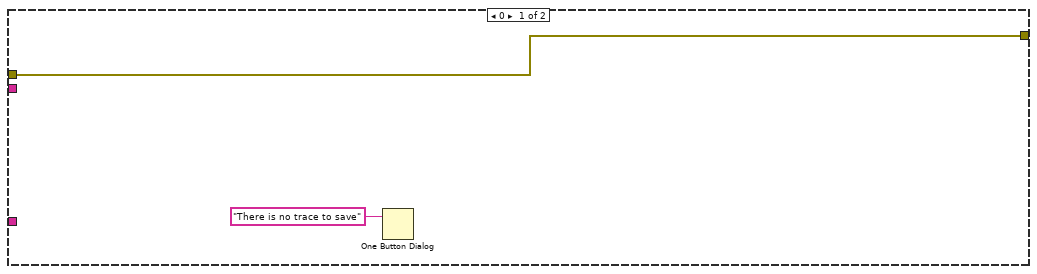
[diagram p18: hidden frame]
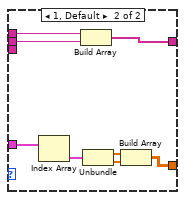
[diagram p19: hidden frame]
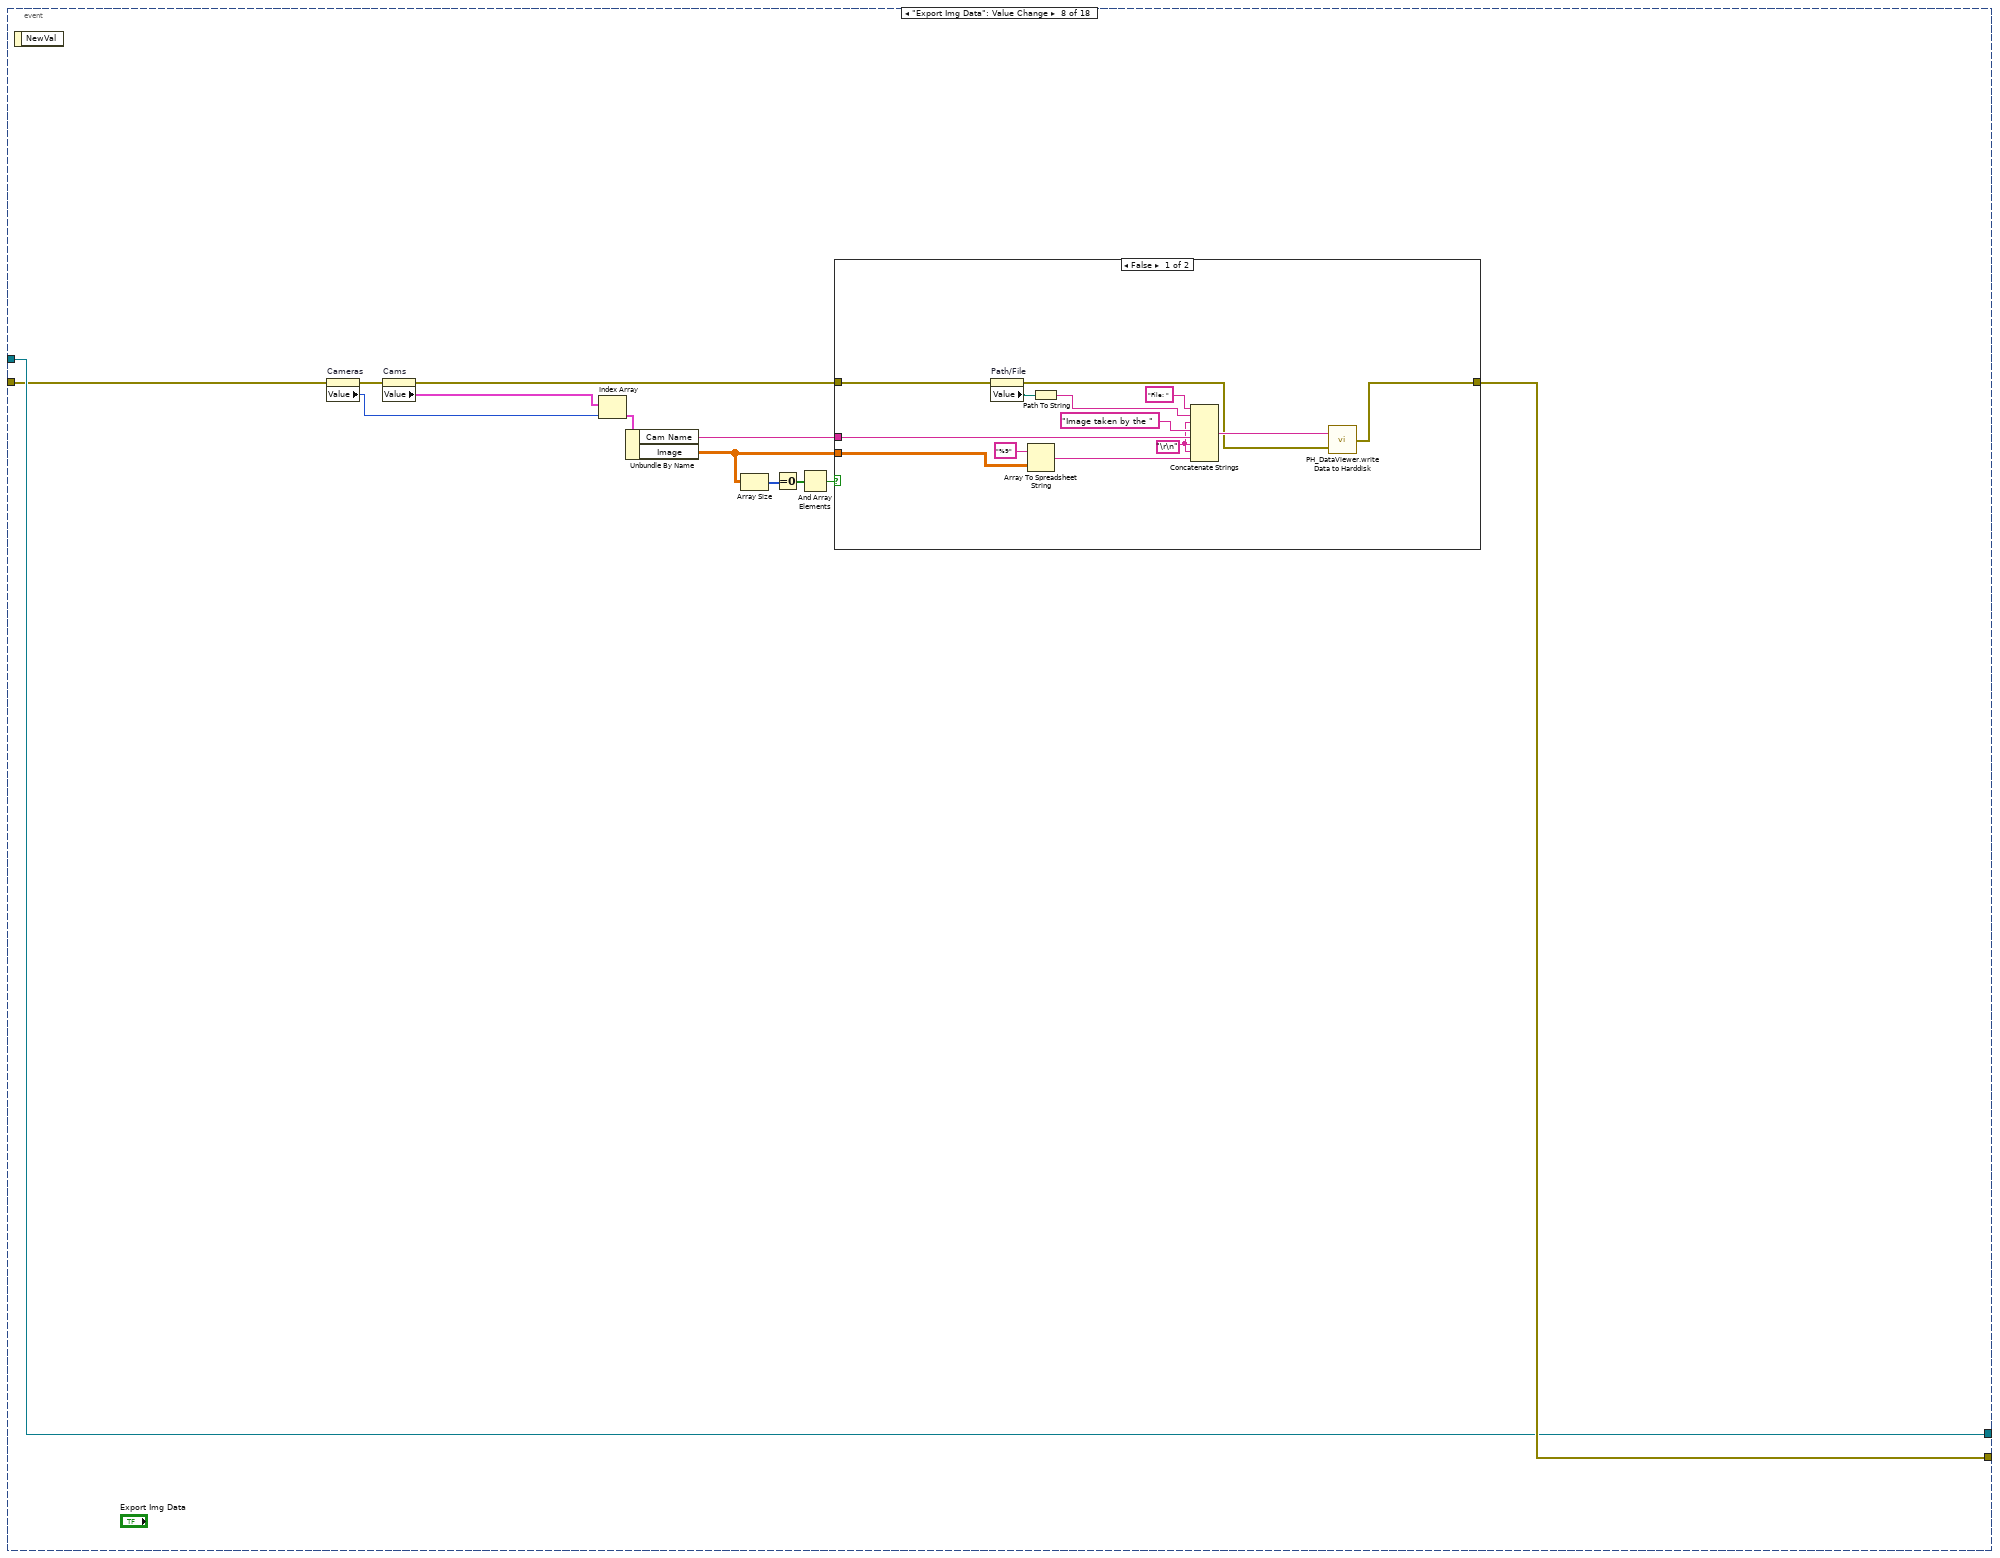
[diagram p20: hidden frame]
diagram:
  n1 = call "PH_DataViewer.get data to modify.vi"("i ref in"="object ref", "ms timeout (10000)"=-1, "error in (no error)"="error in (no error)") -> ("i ref out"=w47:refnum<vi>, "i attribute"=w41:T32, "error out"=w48:errorcluster)  [unwired: 13 in, 1 out]
  n2 = control-ref of="Background Image"() -> (w35:refnum<vi>)
  n3 = control-ref of="Op Image"() -> (w33:refnum<vi>)
  n4 = control-ref of="Bg subtracted"() -> (w34:refnum<vi>)
  n5 = control-ref of="Energy on"() -> (w31:refnum<vi>)
  n6 = control-ref of="Beam Analysis"() -> (w28:refnum<vi>)
  n7 = control-ref of="f rel to major?"() -> (w18:refnum<vi>)
  n8 = control-ref of="Position"() -> (w17:refnum<vi>)
  n9 = control-ref of="Fit Gauss"() -> (w10:refnum<vi>)
  n10 = control-ref of="Calibration data"() -> (w36:refnum<vi>)
  n11 = control-ref of="Cam Settings Operator"() -> (w32:refnum<vi>)
  n12 = control-ref of="exp Energy"() -> (w30:refnum<vi>)
  n13 = control-ref of="Energy"() -> (w29:refnum<vi>)
  n14 = control-ref of="BA: Steps"() -> (w26:refnum<vi>)
  n15 = control-ref of="BA: Factor for ROI"() -> (w25:refnum<vi>)
  n16 = control-ref of="CoG - X"() -> (w24:refnum<vi>)
  n17 = control-ref of="CoG - Y"() -> (w23:refnum<vi>)
  n18 = control-ref of="Maj Diam"() -> (w22:refnum<vi>)
  n19 = control-ref of="Min Diam"() -> (w21:refnum<vi>)
  n20 = control-ref of="f"() -> (w20:refnum<vi>)
  n21 = control-ref of="e"() -> (w19:refnum<vi>)
  n22 = control-ref of="exp - X"() -> (w1:refnum<vi>)
  n23 = control-ref of="exp - Y"() -> (w15:refnum<vi>)
  n24 = control-ref of="M"() -> (w14:refnum<vi>)
  n25 = control-ref of="f 2"() -> (w13:refnum<vi>)
  n26 = control-ref of="D"() -> (w12:refnum<vi>)
  n27 = control-ref of="q"() -> (w11:refnum<vi>)
  n28 = control-ref of="Maj Fit Order"() -> (w9:refnum<vi>)
  n29 = control-ref of="Min Fit Order"() -> (w8:refnum<vi>)
  n30 = control-ref of="Maj FWHM"() -> (w7:refnum<vi>)
  n31 = control-ref of="Min FWHM"() -> (w6:refnum<vi>)
  n32 = control-ref of="Maj 1 %"() -> (w5:refnum<vi>)
  n33 = control-ref of="Min 1 %"() -> (w4:refnum<vi>)
  n34 = control-ref of="Date Operators"() -> (w39:refnum<vi>)
  n35 = control-ref of="Time Operators"() -> (w38:refnum<vi>)
  n36 = control-ref of="Status Cali Data"() -> (w37:refnum<vi>)
  n37 = control-ref of="Analysis Type"() -> (w27:refnum<vi>)
  n38 = control-ref of="Position Type"() -> (w16:refnum<vi>)
  n39 = Bundle By Name(cluster=w41, "Cam Operator GUI Refs.Date Operators"=w39, "Cam Operator GUI Refs.Time Operators"=w38, "Cam Operator GUI Refs.Status Cali Data"=w37, "Cam Operator GUI Refs.Calibration data"=w36, "Cam Operator GUI Refs.Background Image"=w35, "Cam Operator GUI Refs.Bg subtracted"=w34, "Cam Operator GUI Refs.Op Image"=w33, "Cam Operator GUI Refs.Cam Settings Operator"=w32, "Cam Operator GUI Refs.Energy on"=w31, "Cam Operator GUI Refs.exp Energy"=w30, "Cam Operator GUI Refs.Energy"=w29, "Cam Operator GUI Refs.Beam Analysis"=w28, "Cam Operator GUI Refs.Analysis Type"=w27, "Cam Operator GUI Refs.BA: Steps"=w26, "Cam Operator GUI Refs.BA: Factor for ROI"=w25, "Cam Operator GUI Refs.CoG - X"=w24, "Cam Operator GUI Refs.CoG - Y"=w23, "Cam Operator GUI Refs.Maj Diam"=w22, "Cam Operator GUI Refs.Min Diam"=w21, "Cam Operator GUI Refs.Phi"=w20, "Cam Operator GUI Refs.Epsilon"=w19, "Cam Operator GUI Refs.Phi rel to maj"=w18, "Cam Operator GUI Refs.Position"=w17, "Cam Operator GUI Refs.Position Type"=w16, "Cam Operator GUI Refs.exp - X"=w1, "Cam Operator GUI Refs.exp - Y"=w15, "Cam Operator GUI Refs.Magni"=w14, "Cam Operator GUI Refs.Foc Length"=w13, "Cam Operator GUI Refs.Delta"=w12, "Cam Operator GUI Refs.Theta"=w11, "Cam Operator GUI Refs.Fit Gauss"=w10, "Cam Operator GUI Refs.Maj Fit Order"=w9, "Cam Operator GUI Refs.Min Fit Order"=w8, "Cam Operator GUI Refs.Maj FWHM"=w7, "Cam Operator GUI Refs.Min FWHM"=w6, "Cam Operator GUI Refs.Maj 1 %"=w5, "Cam Operator GUI Refs.Min 1 %"=w4) -> (w40:T32)
  n40 = call "PH_DataViewer.set modified data.vi"("i ref in"=w47, "i attribute"=w40, "error in (no error)"=w48) -> ("i ref out"=w45:refnum<vi>, "error out"=w43:errorcluster)  [unwired: 15 in]
  n41 = while {
    tunnel: w45 -> [w51]
    tunnel: [w50] -> w3
    tunnel: w43 -> [w53]
    tunnel: [w52] -> w2
    i -> [w54]
    stop <- w49 stop-if-true
    n42 = event shown="[2] \"Read Data\": Value Change" {
      selector: _ -> [_ _ _ _ _ _ _ _ _ _ _ _ _ _ _ _ _ _]
      dyn-events: _ -> [_ _ _ _ _ _ _ _ _ _ _ _ _ _ _ _ _ _]
      timeout: _ -> [_ _ _ _ _ _ _ _ _ _ _ _ _ _ _ _ _ _]
      tunnel: w51 -> [w55 w61 w137 w288 w313 w387 w451 w514 w542 w570 w612 w630 w632 w666 w680 w697 w755 w769]
      tunnel: w53 -> [w56 w60 w136 w301 w347 w381 w449 w510 w538 w566 w610 w628 w649 w665 w679 w696 w754 w771]
      tunnel: [w56 w59 w129 _ w311 w388 w452 w515 w543 w571 w603 w623 w633 w658 w674 w698 w740 w762] -> w52
      tunnel: [w55 w58 w130 w288 w313 w387 w451 w514 w542 w570 w612 w630 w632 w666 w680 w697 w739 w767] -> w50
      tunnel: [_ "Delete" _ _ _ _ _ _ _ _ _ _ _ _ _ _ _ _] -> w49
      event Timeout {
        n43 = event-data() -> ()  [unwired: 1 in, 2 out]
      }
      event "Delete": Value Change {
        n44 = event-data() -> ()  [unwired: 1 in, 1 out]
        n45 = call "CSObj.open front panel.vi"("i ref in"=w61, "frontPanelOpen"=FALSE ("front panel open"), "error in (no error)"=w60) -> ("i ref out"=w58:refnum<vi>, "error out"=w59:errorcluster)  [unwired: 15 in]
      }
      event "Read Data": Value Change {
        w66 = 0 ("index")
        w78 = 0 ("index")
        w134 = 0 ("index")
        n46 = event-data() -> ()  [unwired: 1 in, 1 out]
        n47 = call "PH_DataViewer.get i attribute.vi"("i ref in"=w137, "error in (no error)"=w136) -> ("i ref out"=w127:refnum<vi>, "i attribute"=w131:T32, "error out"=w91:errorcluster)  [unwired: 15 in]
        n48 = call "PH_DataViewer.Read Data from Disk.vi"("error in"=w91) -> ("Version"=w88:u8, "new file path"=→"Path/File":path, "Data Vers 1"=w87:T37, "Data Vers 2"=w86:T38, "Data Vers 3"=w85:T44, "Data Vers 4"=w73:T45, "error IO"=w89:errorcluster)  [unwired: 12 in]
        n49 = case shown="3" w88 {
          tunnel: w87 -> [w202 w213 w247 w267]
          tunnel: [w201 w225 w243 w264] -> w176
          tunnel: [w200 w224 w242 w263] -> w175
          tunnel: [w199 w212 w246 w266] -> w150
          tunnel: [w198 w223 w244 w265] -> w149
          tunnel: [w197 w222 w237 w258] -> w148
          tunnel: [w196 w221 w236 w257] -> w147
          tunnel: [w195 w220 w235 w256] -> w95
          tunnel: [w194 w219 w238 w259] -> w126
          tunnel: [w193 w218 w233 w254] -> w121
          tunnel: [w192 w217 w234 w255] -> w120
          tunnel: [w191 w216 w241 w262] -> w116
          tunnel: [w190 w215 w240 w261] -> w115
          tunnel: w86 -> [w189 w214 _ _]
          tunnel: [w188 w211 w239 w260] -> w98
          tunnel: [w187 w210 w232 w253] -> w93
          tunnel: [w186 w209 w231 w252] -> w94
          tunnel: [w183 TRUE w229 w248] -> w92
          tunnel: w85 -> [w185 w207 w245 _]
          tunnel: [w184 w206 w230 w251] -> w80
          tunnel: [w183 w205 w229 w248] -> w74
          tunnel: w73 -> [w182 w204 w227 w250]
          tunnel: [w181 w203 w226 w249] -> w69
          tunnel: [w183 w205 FALSE w248] -> w65
          frame Default {
            w183 = FALSE
            n50 = Unbundle By Name(w202) -> ("Triggers"=w198:T25[], "Black Boxes"=w201:T31[], "Calorimeters"=w200:T33[], "Current Meas'"=w191:T35[], "Powermeters"=w190:T12[], "PP PUs"=w199:T11[], "BNC555s"=w194:T27, "Chillers"=w197:T29[], "Mercury Monitors"=w196:T36[], "Vac Controls"=w195:T30[], "Cams"=w192:T9[], "Img Operators"=w193:T5[])
            n51 = Unbundle By Name(w185) -> ("Backreflection Meas"=w184:T2[])
            n52 = Unbundle By Name(w189) -> ("PP PUs"=w188:T3[], "SRDG535s"=w187:T39[], "Sequencer Data"=w186:T14)
            n53 = Unbundle By Name(w182) -> ("OO Spectrometer"=w181:T1[])
          }
          frame 2 {
            w205 = FALSE
            n54 = Unbundle By Name(w213) -> ("PP PUs"=w212:T11[])
            n55 = Unbundle By Name(w214) -> ("Triggers"=w223:T25[], "Black Boxes"=w225:T31[], "Calorimeters"=w224:T33[], "Current Meas'"=w216:T35[], "Powermeters"=w215:T12[], "PP PUs"=w211:T3[], "BNC555s"=w219:T27, "Chillers"=w222:T29[], "Mercury Monitors"=w221:T36[], "Vac Controls"=w220:T30[], "Cams"=w217:T9[], "Img Operators"=w218:T5[], "SRDG535s"=w210:T39[], "Sequencer Data"=w209:T14)
            n56 = Unbundle By Name(w207) -> ("Backreflection Meas"=w206:T2[])
            n57 = Unbundle By Name(w204) -> ("OO Spectrometer"=w203:T1[])
          }
          frame 3 {
            w229 = TRUE
            n58 = Unbundle By Name(w245) -> ("Triggers"=w244:T25[], "Black Boxes"=w243:T31[], "Calorimeters"=w242:T33[], "Current Meas'"=w241:T35[], "Powermeters"=w240:T12[], "PP PUs"=w239:T3[], "BNC555s"=w238:T27, "Chillers"=w237:T29[], "Mercury Monitors"=w236:T36[], "Vac Controls"=w235:T30[], "Cams"=w234:T9[], "Img Operators"=w233:T5[], "SRDG535s"=w232:T39[], "Sequencer Data"=w231:T14, "Backreflection Meas"=w230:T2[])
            n59 = Unbundle By Name(w247) -> ("PP PUs"=w246:T11[])
            n60 = Unbundle By Name(w227) -> ("OO Spectrometer"=w226:T1[])
          }
          frame 4 {
            w248 = TRUE
            n61 = Unbundle By Name(w250) -> ("Triggers"=w265:T25[], "Black Boxes"=w264:T31[], "Calorimeters"=w263:T33[], "Current Meas'"=w262:T35[], "Powermeters"=w261:T12[], "PP PUs"=w260:T3[], "BNC555s"=w259:T27, "Chillers"=w258:T29[], "Mercury Monitors"=w257:T36[], "Vac Controls"=w256:T30[], "Cams"=w255:T9[], "Img Operators"=w254:T5[], "SRDG535s"=w253:T39[], "Sequencer Data"=w252:T14, "Backreflection Meas"=w251:T2[], "OO Spectrometer"=w249:T1[])
            n62 = Unbundle By Name(w267) -> ("PP PUs"=w266:T11[])
          }
        }
        "Black Boxes" <- w176
        "Powermeters" <- w115
        "Triggers" <- w149
        "Vac Controls" <- w95
        "Chillers" <- w148
        "Cams" <- w120
        "Img Operators" <- w121
        "BNC555s" <- w126
        "Backreflection Meas" <- w80
        "OO Spectrometer" <- w69
        n63 = Unbundle By Name(w131) -> ("Images.CAM"=w132:cluster{string, u32})
        n64 = call <vilib>:"IMAQ Image Cluster to Image Datatype.vi"("Image"=w132) -> ("Image (dup)"=w123:T21)
        n65 = Index Array(array=w121, index=0) -> (element=w125:T5)
        n66 = Unbundle By Name(w125) -> ("Trace Analysis.on"=w122:bool, "Trace Analysis.Traces"=w124:T46)
        n67 = call "PH_DataViewer.set Img Op GUI elements.vi"("i ref in"=w127, "Img Operator Data"=w125, "error in (no error)"=w89) -> ("i ref out"=w130:refnum<vi>, "error out"=w129:errorcluster)  [unwired: 15 in]
        n68 = case shown="True" w122 {
          tunnel: w124 -> [_ w283]
          frame False {
            w268 = cluster{"Index":sgl[], dbl[]}[] [] ("Major Trace")
            "Major Trace" <- w268
            "Minor Trace" <- w268
          }
          frame True {
            n69 = Index Array(array=w283) -> (element #1=w282:T47, element #2=w275:T47)  [unwired: 2 in]
            n70 = Unbundle By Name(w282) -> ("XScaleName"=w281:string, "Y Scale Minimum"=w280:sgl, "Y Scale Maximum"=w279:sgl, "X Scale Minimum"=w278:sgl, "X Scale Maximum"=w277:sgl, "Traces"=w276:cluster{"Index":sgl[], "Trace":dbl[]}[])
            n71 = property on="Major Trace" class="XYGraph (strict)"("X Scale.Name Label.Text"=w281, "Y Scale.Range:Minimum"=w280, "Y Scale.Range:Maximum"=w279, "X Scale.Range:Minimum"=w278, "X Scale.Range:Maximum"=w277, "Value"=w276) -> ()  [unwired: 2 in, 2 out]
            n72 = Unbundle By Name(w275) -> ("XScaleName"=w274:string, "Y Scale Minimum"=w273:sgl, "Y Scale Maximum"=w272:sgl, "X Scale Minimum"=w271:sgl, "X Scale Maximum"=w270:sgl, "Traces"=w269:cluster{"Index":sgl[], "Trace":dbl[]}[])
            n73 = property on="Minor Trace" class="XYGraph (strict)"("X Scale.Name Label.Text"=w274, "Y Scale.Range:Minimum"=w273, "Y Scale.Range:Maximum"=w272, "X Scale.Range:Minimum"=w271, "X Scale.Range:Maximum"=w270, "Value"=w269) -> ()  [unwired: 2 in, 2 out]
          }
        }
        n74 = Index Array(array=w69, index=w66) -> (element=w72:T1)
        n75 = Index Array(array=w80, index=w78) -> (element=w83:T2)
        n76 = Unbundle By Name(w72) -> ("Date"=w71:string, "Time"=w70:string, "Wavelength Bins"=w64:dbl[], "Spectrum by Pixels"=w63:dbl[])
        n77 = Unbundle By Name(w83) -> ("Snapshot: Date"=w75:string, "Snapshot: Time"=w76:string, "Waveform Data.Waveform Array"=w82:dbl[], "Waveform Data.X Increment"=w81:dbl)
        n78 = for {
          tunnel: w69 -> [w178] mode=indexing
          tunnel: [w177] -> w68 mode=indexing
          n79 = Unbundle By Name(w178) -> ("Instance"=w177:string)
        }
        n80 = for {
          tunnel: w120 -> [w287] mode=indexing
          tunnel: [w286] -> w145 mode=indexing
          n81 = Unbundle By Name(w287) -> ("Cam Name"=w286:string)
        }
        n82 = Index Array(array=w120, index=0) -> (element=w143:T9)
        n83 = for {
          tunnel: w121 -> [w285] mode=indexing
          tunnel: [w284] -> w133 mode=indexing
          n84 = Unbundle By Name(w285) -> ("Instance"=w284:string)
        }
        n85 = Unbundle By Name(w143) -> ("Image"=w135:sgl[][], "Img taken: Date"=→"Date Cams":string, "Img Taken: Time"=→"Time Cams":string, "Cam Settings"=→"Cam Settings":T10, "Cam.Trigger"=→"Cam Trigger":T19)
        n86 = for {
          tunnel: w80 -> [w180] mode=indexing
          tunnel: [w179] -> w79 mode=indexing
          n87 = Unbundle By Name(w180) -> ("Instance"=w179:string)
        }
        n88 = call "PH_BackreflectionMeas.create waveform.vi"("dt"=w81, "Y-Data"=w82) -> ("waveform out"=w84:waveform(dbl))
        n89 = Not Equal?(x=w88, y=u8 2) -> (x != y?=w96:bool)
        n90 = call "PH_DataViewer.set Calorimeter GUI elements.vi"("Calorimeters"=w175, "Version"=w88) -> ("PH Calorimeter Device Config"=→"PH Calorimeter Device Config":T34, "Energy [J]"=→"Energy [J]":dbl, "Graph Data"=→"Graph":cluster{"Raw Data":dbl[], "Raw Data":dbl[]}, "Taken + Calc: Date"=→"Date Calo":string, "Taken + Calc: Time"=→"Time Calo":string)  [unwired: 9 in]
        n91 = call "PH_DataViewer.set Current Meas GUI Elements.vi"("Current Meas'"=w116, "Version"=w88) -> ("Snapshot: Date"=→"Date Current Meas":string, "Data"=→"Current Meas Data":waveform(dbl)[][], "Snapshot: Time"=→"Time Current Meas":string, "Ignore Timestamp"=w164:bool, "Power Unit List"=w168:string[], "index"=w163:i32, "PU Name"=w167:string, "Graph Data"=w165:waveform(dbl)[], "X Scale.Format & Precision:Precision"=w169:u8, "index of element"=w166:i32)  [unwired: 8 in]
        n92 = call "PH_DataViewer.set Powermeter GUI elements.vi"("Powermeters"=w115, "Version"=w88) -> ("Instances"=w114:string[], "Status"=→"Status Powermeter":u32, "index"=w113:i32, "Trigger Level"=→"Trigger Level":dbl, "Snapshot: Date"=→"Date Powermeter":string, "Snapshot: Time"=→"Time Powermeter":string, "Serial Number"=→"Serial Number":string, "Current Value"=→"Current Value":dbl, "Current Value Unit"=→"Unit":string, "Scaling Factor"=→"Scaling Factor":dbl)  [unwired: 8 in]
        n93 = call "PH_DataViewer.set PU GUI Elements.vi"("index"=0, "PP PUs Vers 1"=w150, "PP PUs Vers 2"=w98, "Version"=w88) -> ("Instances"=w102:string[], "index"=w103:i32, "PP PUs"=→"PP PUs":T11[], "Snapshot: Date before Shot"=→"Date PU before Shot":string, "State after Shot"=→"State after Shot":T4, "Snapshot: Time before Shot"=→"Time PU before Shot":string, "PU in use after Shot"=→"in use after Shot":bool, "PU in use before Shot"=→"in use before Shot":bool, "Snapshot: Time after Shot"=→"Time PU after Shot":string, "State before Shot"=→"State before Shot":T4, "Waiting Time over?"=→"Waiting Time over":bool, "Voltage [V]"=→"Voltage [V]":dbl, "Delay [s]"=w100:dbl, "Gate Gen Channel"=w99:string, "Timeout SM"=→"Timeout SM":string, "Time betweeen Shots [Min]"=→"Waiting Time [Min]":dbl, "Snapshot: Date after Shot"=→"Date PU after Shot":string)  [unwired: 7 in]
        n94 = Index Array(array=w147) -> (element=→"Mercury Monitor":T36)  [unwired: 1 in]
        n95 = call "IMAQ ArrayToImage"("Image Pixels (Float)"=w135, "Image"=w123) -> ("Image Out"=→"Cam Image":T21)  [unwired: 8 in, 1 out]
        n96 = Bundle("Wavelength Bins"=w64, "Spectrum by Pixels"=w63) -> (w67:T48)  [unwired: 1 in]
        n97 = Build Array(w84) -> (w77:waveform(dbl)[])
        n98 = property on="SRDGs" class="Arr (strict)"("Value"=w93, "Visible"=w92) -> ()  [unwired: 2 in, 2 out]
        n99 = property on="Sequencer Data" class="Clust (strict)"("Value"=w94, "Visible"=w92) -> ()  [unwired: 2 in, 2 out]
        n100 = property on="Date BRM" class="Str"("Value"=w75, "Visible"=w74) -> ()  [unwired: 2 in, 2 out]
        n101 = property on="Time BRM" class="Str"("Value"=w76, "Visible"=w74) -> ()  [unwired: 2 in, 2 out]
        n102 = property on="BRM Graph" class="WFGraph (strict)"("Value"=w77, "Visible"=w74) -> ()  [unwired: 2 in, 2 out]
        n103 = property on="Export Data BRM" class="Bool"("Visible"=w74) -> ()  [unwired: 2 in, 2 out]
        n104 = property on="Date OO Spectro" class="Str"("Value"=w71, "Visible"=w65) -> ()  [unwired: 2 in, 2 out]
        n105 = property on="Time OO Spectro" class="Str"("Value"=w70, "Visible"=w65) -> ()  [unwired: 2 in, 2 out]
        n106 = property on="OO Spectrum" class="XYGraph (strict)"("Value"=w67, "Visible"=w65) -> ()  [unwired: 2 in, 2 out]
        n107 = property on="Export OO Spectro Data" class="Bool"("Visible"=w65) -> ()  [unwired: 2 in, 2 out]
        n108 = property on="Backreflection Measurement" class="Ring (strict)"("Value"=w78, "Strings []"=w79, "Visible"=w74) -> ()  [unwired: 2 in, 2 out]
        n109 = property on="OO Spectrometer Instancelist" class="Ring (strict)"("Value"=w66, "Strings []"=w68, "Visible"=w65) -> ()  [unwired: 2 in, 2 out]
        n110 = property on="Delay [s]" class="DigNum (strict)"("Value"=w100, "Visible"=w96) -> ()  [unwired: 2 in, 2 out]
        n111 = property on="Gate Gen Chan" class="Str"("Value"=w99, "Visible"=w96) -> ()  [unwired: 2 in, 2 out]
        n112 = property on="Cameras" class="Ring (strict)"("Strings []"=w145, "Value"=w134) -> ()  [unwired: 2 in, 2 out]
        n113 = property on="Operators" class="Ring (strict)"("Strings []"=w133, "Value"=w134) -> ()  [unwired: 2 in, 2 out]
        n114 = property on="Power Unit CM" class="Ring (strict)"("Strings []"=w168, "Value"=w163) -> ()  [unwired: 2 in, 2 out]
        n115 = property on="Powermeter" class="Ring (strict)"("Strings []"=w114, "Value"=w113) -> ()  [unwired: 2 in, 2 out]
        n116 = property on="Power Unit" class="Ring (strict)"("Strings []"=w102, "Value"=w103) -> ()  [unwired: 2 in, 2 out]
        n117 = property on="current meas data indicator" class="WFGraph (strict)"("Caption.Text"=w167, "Value"=w165, "X Scale.Format & Precision:Precision"=w169, "Legend:Plots Shown"=w166, "Ignore Timestamp"=w164) -> ()  [unwired: 2 in, 2 out]
      }
      event "Power Unit CM": Value Change {
        n118 = event-data() -> ("NewVal"=w293:u16)  [unwired: 1 in]
        n119 = property on="Current Meas Data" class="Arr (strict)"(error in=w301) -> (error out=w300:errorcluster, "Value"=w299:waveform(dbl)[][])  [unwired: 1 in, 1 out]
        n120 = Index Array(array=w299, index (row)=w293) -> (element=w291:waveform(dbl)[])  [unwired: 1 in]
        n121 = property on="Power Unit CM" class="Ring (strict)"() -> ("Strings []"=w294:string[])  [unwired: 2 in, 2 out]
        n122 = for {
          tunnel: w291 -> [w309] mode=indexing
          tunnel: [w306] -> w296 mode=indexing
          n123 = Unbundle By Name(w309) -> ("dt"=w308:dbl)
          n124 = Equal?(x=w308, y=0.0) -> (x = y?=w306:bool)
        }
        n125 = Index Array(array=w294, index=w293) -> (element=w292:string)
        n126 = Search 1D Array(1D array=w296, element=TRUE) -> (index of element=w290:i32)  [unwired: 1 in]
        n127 = case shown="Default" w290 {
          selector: w290 -> [w302 _ _]
          tunnel: w291 -> [_ _ w305]
          tunnel: [w302 1 ("index of element") w304] -> w289
          frame Default {
          }
          frame 0 {
          }
          frame -1 {
            n128 = Array Size(array=w305) -> (size(s)=w304:i32)
          }
        }
        n129 = property on="current meas data indicator" class="WFGraph (strict)"(error in=w300, "Value"=w291, "Ignore Timestamp"=TRUE, "X Scale.Format & Precision:Precision"=u8 6, "Legend:Plots Shown"=w289, "Caption.Text"=w292) -> ()  [unwired: 1 in, 2 out]
      }
      event "Export Current Meas Data": Value Change {
        w327 = "\r\n"
        n130 = event-data() -> ()  [unwired: 1 in, 1 out]
        n131 = property on="Current Meas Data" class="Arr (strict)"(error in=w347) -> (error out=w315:errorcluster, "Value"=w346:waveform(dbl)[][])  [unwired: 1 in, 1 out]
        n132 = property on="Power Unit CM" class="Ring (strict)"(error in=w315) -> (error out=w314:errorcluster, "Value"=w345:u16)  [unwired: 1 in, 1 out]
        n133 = Index Array(array=w346, index (row)=w345) -> (element=w341:waveform(dbl)[])  [unwired: 1 in]
        n134 = for {
          tunnel: w341 -> [w374] mode=indexing
          tunnel: [w371] -> w344 mode=indexing
          n135 = Unbundle By Name(w374) -> ("dt"=w373:dbl)
          n136 = Equal?(x=w373, y=0.0) -> (x = y?=w371:bool)
        }
        n137 = Search 1D Array(1D array=w344, element=TRUE) -> (index of element=w342:i32)  [unwired: 1 in]
        n138 = property on="Power Unit CM" class="Ring (strict)"(error in=w314) -> (error out=w316:errorcluster, "Strings []"=w332:string[], "Value"=w331:u16)  [unwired: 1 in, 1 out]
        n139 = case shown="Default" w342 {
          selector: w342 -> [w366 _ _]
          tunnel: w341 -> [w367 _ w370]
          tunnel: [w365 "Empty" w370] -> w323
          frame Default {
            n140 = for {
              N: w366 -> [_]
              tunnel: w367 -> [w368] mode=indexing
              tunnel: [w368] -> w365 mode=indexing
            }
          }
          frame 0 {
          }
          frame -1 {
          }
        }
        n141 = Index Array(array=w332, index=w331) -> (element=w330:string)
        n142 = Index Array(array=w323) -> (element=w340:waveform(dbl))  [unwired: 1 in]
        n143 = property on="Path/File" class="Path"(error in=w316) -> (error out=w312:errorcluster, "Value"=w326:path)  [unwired: 1 in, 1 out]
        n144 = for {
          tunnel: w323 -> [w359] mode=indexing
          tunnel: [w348] -> w320 mode=indexing
          w353 = ""
          n145 = Unbundle By Name(w359) -> ("attributes"=w355:variant)
          n146 = Get Variant Attribute(Variant=w355, name="NI_ChannelName") -> (value=w357:variant)  [unwired: 2 in, 3 out]
          n147 = Get Variant Attribute(Variant=w355, name="NI_UnitDescription") -> (value=w354:variant)  [unwired: 2 in, 3 out]
          n148 = Variant To Data(type=w353, Variant=w354) -> (data=w350:string)  [unwired: 1 in, 1 out]
          n149 = Variant To Data(type=w353, Variant=w357) -> (data=w352:string)  [unwired: 1 in, 1 out]
          n150 = Concatenate Strings(w352, " [" ("string"), w350, "]" ("string")) -> (w348:string)
        }
        n151 = Unbundle By Name(w340) -> ("Y"=w335:dbl[], "dt"=w339:dbl)
        n152 = Path To String(path=w326) -> (string=w325:string)
        n153 = for {
          tunnel: w339 -> [w363]
          tunnel: [w362] -> w338 mode=indexing
          tunnel: w335 -> [_] mode=indexing
          i -> [w364]
          n154 = Multiply(x=w364, y=w363) -> (x*y=w362:dbl)
        }
        n155 = for {
          tunnel: w323 -> [w361] mode=indexing
          tunnel: [w360] -> w337 mode=indexing
          n156 = Unbundle By Name(w361) -> ("Y"=w360:dbl[])
        }
        n157 = Build Array (concatenate)(w338, w337) -> (w336:dbl[][])
        n158 = Transpose 2D Array(2D array=w336) -> (transposed array=w334:dbl[][])
        n159 = Array To Spreadsheet String(array=w334, 3:"%9" ("format string")) -> (spreadsheet string=w329:string)  [unwired: 1 in]
        n160 = Insert Into Array(array=w320, index=0, new element="Time [s]" ("new element/subarray")) -> (w321:string[])
        n161 = Array To Spreadsheet String(array=w321, 3:"%s" ("format string")) -> (spreadsheet string=w318:string)  [unwired: 1 in]
        n162 = Concatenate Strings("File: " ("string"), w325, w327, "Current Data of the ", w330, w327, w327, w318, w329) -> (w310:string)
        n163 = call "PH_DataViewer.write Data to Harddisk.vi"("error in"=w312, "String"=w310) -> ("error out"=w311:errorcluster)
      }
      event "Export Maj Trace": Value Change {
        n164 = event-data() -> ()  [unwired: 1 in, 1 out]
        n165 = property on="Operators" class="Ring (strict)"(error in=w381) -> (error out=w380:errorcluster, "Value"=w378:u16)  [unwired: 1 in, 1 out]
        n166 = property on="Img Operators" class="Arr (strict)"(error in=w380) -> (error out=w382:errorcluster, "Value"=w379:T5[])  [unwired: 1 in, 1 out]
        n167 = Index Array(array=w379, index=w378) -> (element=w377:T5)
        n168 = Unbundle By Name(w377) -> ("Trace Analysis.Maj Fit Order"=w375:i32)
        n169 = property on="Major Trace" class="XYGraph (strict)"(error in=w382) -> (error out=w386:errorcluster, "X Scale.Name Label.Text"=w384:string, "Value"=w383:cluster{"Index":sgl[], dbl[]}[])  [unwired: 1 in, 1 out]
        n170 = Number To Decimal String(number=w375) -> (decimal integer string=w376:string)  [unwired: 1 in]
        n171 = Array Size(array=w383) -> (size(s)=w385:i32)
        n172 = case shown="Default" w385 {
          selector: w385 -> [_ w395]
          tunnel: [w389 w391] -> w388
          tunnel: w386 -> [w389 w407]
          tunnel: w384 -> [_ w394]
          tunnel: w383 -> [_ w402]
          tunnel: w376 -> [_ w397]
          frame 0 {
            n173 = One Button Dialog(message="There is no trace to save") -> ()  [unwired: 1 in, 1 out]
          }
          frame Default {
            w416 = "\r\n"
            n174 = property on="Operators" class="Ring (strict)"(error in=w407) -> (error out=w410:errorcluster, "Strings []"=w408:string[], "Value"=w409:u16)  [unwired: 1 in, 1 out]
            n175 = Concatenate Strings("Gauss Fit [" ("element"), w397, " Order]" ("string")) -> (w398:string)
            n176 = Index Array(array=w408, index=w409) -> (element=w418:string)
            n177 = case shown="1, Default" w395 {
              tunnel: w394 -> [w430 w438]
              tunnel: [w429 w437] -> w406
              tunnel: [w428 w436] -> w404
              tunnel: w402 -> [w421 w432]
              tunnel: "Trace" ("element") -> [w420 w431]
              tunnel: w398 -> [w419 _]
              frame 2 {
                n178 = Index Array(array=w421) -> (element #1=w426:cluster{"Index":sgl[], dbl[]}, element #2=w427:cluster{"Index":sgl[], dbl[]})  [unwired: 2 in]
                n179 = Build Array(w430, w420, w419) -> (w429:string[])
                n180 = Unbundle(w426) -> ("Index"=w425:sgl[], w424:dbl[])
                n181 = Unbundle(w427) -> ("Index"=w423:sgl[], w422:dbl[])
                n182 = Build Array(w425, w424, w423, w422) -> (w428:dbl[][])
              }
              frame 1, Default {
                n183 = Index Array(array=w432) -> (element=w435:cluster{"Index":sgl[], dbl[]})  [unwired: 1 in]
                n184 = Build Array(w438, w431) -> (w437:string[])
                n185 = Unbundle(w435) -> ("Index"=w434:sgl[], w433:dbl[])
                n186 = Build Array(w434, w433) -> (w436:dbl[][])
              }
            }
            n187 = property on="Path/File" class="Path"(error in=w410) -> (error out=w392:errorcluster, "Value"=w415:path)  [unwired: 1 in, 1 out]
            n188 = Path To String(path=w415) -> (string=w414:string)
            n189 = Transpose 2D Array(2D array=w404) -> (transposed array=w403:dbl[][])
            n190 = Array To Spreadsheet String(array=w406, 3:"%s" ("format string")) -> (spreadsheet string=w411:string)  [unwired: 1 in]
            n191 = Array To Spreadsheet String(array=w403, 3:"%9" ("format string")) -> (spreadsheet string=w401:string)  [unwired: 1 in]
            n192 = Concatenate Strings("File: " ("string"), w414, w416, "Major trace of ", w418, w416, w416, w411, w401) -> (w393:string)
            n193 = call "PH_DataViewer.write Data to Harddisk.vi"("error in"=w392, "String"=w393) -> ("error out"=w391:errorcluster)
          }
        }
      }
      event "Export Min Trace": Value Change {
        n194 = event-data() -> ()  [unwired: 1 in, 1 out]
        n195 = property on="Operators" class="Ring (strict)"(error in=w449) -> (error out=w448:errorcluster, "Value"=w446:u16)  [unwired: 1 in, 1 out]
        n196 = property on="Img Operators" class="Arr (strict)"(error in=w448) -> (error out=w442:errorcluster, "Value"=w447:T5[])  [unwired: 1 in, 1 out]
        n197 = Index Array(array=w447, index=w446) -> (element=w445:T5)
        n198 = Unbundle By Name(w445) -> ("Trace Analysis.Min Fit Order"=w443:i32)
        n199 = property on="Minor Trace" class="XYGraph (strict)"(error in=w442) -> (error out=w441:errorcluster, "X Scale.Name Label.Text"=w440:string, "Value"=w439:cluster{"Index":sgl[], dbl[]}[])  [unwired: 1 in, 1 out]
        n200 = Number To Decimal String(number=w443) -> (decimal integer string=w444:string)  [unwired: 1 in]
        n201 = Array Size(array=w439) -> (size(s)=w450:i32)
        n202 = case shown="Default" w450 {
          selector: w450 -> [_ w459]
          tunnel: [w453 w456] -> w452
          tunnel: w441 -> [w453 w471]
          tunnel: w440 -> [_ w458]
          tunnel: w439 -> [_ w466]
          tunnel: w444 -> [_ w461]
          frame 0 {
            n203 = One Button Dialog(message="There is no trace to save") -> ()  [unwired: 1 in, 1 out]
          }
          frame Default {
            w480 = "\r\n"
            n204 = property on="Operators" class="Ring (strict)"(error in=w471) -> (error out=w474:errorcluster, "Strings []"=w472:string[], "Value"=w473:u16)  [unwired: 1 in, 1 out]
            n205 = Concatenate Strings("Gauss Fit [" ("element"), w461, " Order]" ("string")) -> (w462:string)
            n206 = Index Array(array=w472, index=w473) -> (element=w482:string)
            n207 = case shown="2" w459 {
              tunnel: w458 -> [w494 w502]
              tunnel: [w493 w501] -> w470
              tunnel: [w492 w500] -> w468
              tunnel: w466 -> [w485 w496]
              tunnel: "Trace" ("element") -> [w484 w495]
              tunnel: w462 -> [w483 _]
              frame 2 {
                n208 = Index Array(array=w485) -> (element #1=w490:cluster{"Index":sgl[], dbl[]}, element #2=w491:cluster{"Index":sgl[], dbl[]})  [unwired: 2 in]
                n209 = Build Array(w494, w484, w483) -> (w493:string[])
                n210 = Unbundle(w490) -> ("Index"=w489:sgl[], w488:dbl[])
                n211 = Unbundle(w491) -> ("Index"=w487:sgl[], w486:dbl[])
                n212 = Build Array(w489, w488, w487, w486) -> (w492:dbl[][])
              }
              frame 1, Default {
                n213 = Index Array(array=w496) -> (element=w499:cluster{"Index":sgl[], dbl[]})  [unwired: 1 in]
                n214 = Build Array(w502, w495) -> (w501:string[])
                n215 = Unbundle(w499) -> ("Index"=w498:sgl[], w497:dbl[])
                n216 = Build Array(w498, w497) -> (w500:dbl[][])
              }
            }
            n217 = property on="Path/File" class="Path"(error in=w474) -> (error out=w457:errorcluster, "Value"=w479:path)  [unwired: 1 in, 1 out]
            n218 = Path To String(path=w479) -> (string=w478:string)
            n219 = Transpose 2D Array(2D array=w468) -> (transposed array=w467:dbl[][])
            n220 = Array To Spreadsheet String(array=w470, 3:"%s" ("format string")) -> (spreadsheet string=w475:string)  [unwired: 1 in]
            n221 = Array To Spreadsheet String(array=w467, 3:"%9" ("format string")) -> (spreadsheet string=w465:string)  [unwired: 1 in]
            n222 = Concatenate Strings("File: " ("string"), w478, w480, "Minor trace of ", w482, w480, w480, w475, w465) -> (w455:string)
            n223 = call "PH_DataViewer.write Data to Harddisk.vi"("error in"=w457, "String"=w455) -> ("error out"=w456:errorcluster)
          }
        }
      }
      event "Export Img Data": Value Change {
        n224 = event-data() -> ()  [unwired: 1 in, 1 out]
        n225 = property on="Cameras" class="Ring (strict)"(error in=w510) -> (error out=w511:errorcluster, "Value"=w509:u16)  [unwired: 1 in, 1 out]
        n226 = property on="Cams" class="Arr (strict)"(error in=w511) -> (error out=w512:errorcluster, "Value"=w513:T49[])  [unwired: 1 in, 1 out]
        n227 = Index Array(array=w513, index=w509) -> (element=w508:T49)
        n228 = Unbundle By Name(w508) -> ("Cam Name"=w507:string, "Image"=w504:sgl[][])
        n229 = Array Size(array=w504) -> (size(s)=w506:i32[])
        n230 = Equal To 0?(x=w506) -> (x = 0?=w505:bool[])
        n231 = And Array Elements(Boolean array=w505) -> (logical AND=w503:bool)
        n232 = case shown="False" w503 {
          tunnel: [w528 w530] -> w515
          tunnel: w512 -> [w527 w530]
          tunnel: w507 -> [w526 _]
          tunnel: w504 -> [w525 _]
          frame False {
            w523 = "\r\n"
            n233 = property on="Path/File" class="Path"(error in=w527) -> (error out=w516:errorcluster, "Value"=w522:path)  [unwired: 1 in, 1 out]
            n234 = Array To Spreadsheet String(array=w525, 3:"%9" ("format string")) -> (spreadsheet string=w519:string)  [unwired: 1 in]
            n235 = Path To String(path=w522) -> (string=w521:string)
            n236 = Concatenate Strings("File: " ("string"), w521, w523, "Image taken by the ", w526, w523, w523, w519) -> (w517:string)
            n237 = call "PH_DataViewer.write Data to Harddisk.vi"("error in"=w516, "String"=w517) -> ("error out"=w528:errorcluster)
          }
          frame True {
            n238 = One Button Dialog(message="There is no image to save!") -> ()  [unwired: 1 in, 1 out]
          }
        }
      }
      event "Export Op Img": Value Change {
        n239 = event-data() -> ()  [unwired: 1 in, 1 out]
        n240 = property on="Operators" class="Ring (strict)"(error in=w538) -> (error out=w537:errorcluster, "Value"=w539:u16)  [unwired: 1 in, 1 out]
        n241 = property on="Img Operators" class="Arr (strict)"(error in=w537) -> (error out=w536:errorcluster, "Value"=w535:T5[])  [unwired: 1 in, 1 out]
        n242 = Index Array(array=w535, index=w539) -> (element=w541:T5)
        n243 = Unbundle By Name(w541) -> ("Instance"=w540:string, "Image"=w534:dbl[][])
        n244 = Array Size(array=w534) -> (size(s)=w533:i32[])
        n245 = Equal To 0?(x=w533) -> (x = 0?=w532:bool[])
        n246 = And Array Elements(Boolean array=w532) -> (logical AND=w531:bool)
        n247 = case shown="False" w531 {
          tunnel: [w556 w558] -> w543
          tunnel: w540 -> [w555 _]
          tunnel: w536 -> [w554 w558]
          tunnel: w534 -> [w553 _]
          frame False {
            w551 = "\r\n"
            n248 = property on="Path/File" class="Path"(error in=w554) -> (error out=w544:errorcluster, "Value"=w550:path)  [unwired: 1 in, 1 out]
            n249 = Path To String(path=w550) -> (string=w549:string)
            n250 = Array To Spreadsheet String(array=w553, 3:"%9" ("format string")) -> (spreadsheet string=w547:string)  [unwired: 1 in]
            n251 = Concatenate Strings("File: " ("string"), w549, w551, "Image taken by the ", w555, w551, w551, w547) -> (w545:string)
            n252 = call "PH_DataViewer.write Data to Harddisk.vi"("error in"=w544, "String"=w545) -> ("error out"=w556:errorcluster)
          }
          frame True {
            n253 = One Button Dialog(message="There is no image to save!") -> ()  [unwired: 1 in, 1 out]
          }
        }
      }
      event "Export BG Img": Value Change {
        n254 = event-data() -> ()  [unwired: 1 in, 1 out]
        n255 = property on="Operators" class="Ring (strict)"(error in=w566) -> (error out=w565:errorcluster, "Value"=w567:u16)  [unwired: 1 in, 1 out]
        n256 = property on="Img Operators" class="Arr (strict)"(error in=w565) -> (error out=w564:errorcluster, "Value"=w563:T5[])  [unwired: 1 in, 1 out]
        n257 = Index Array(array=w563, index=w567) -> (element=w569:T5)
        n258 = Unbundle By Name(w569) -> ("Instance"=w568:string, "Calibration.Calibration data - Version 1.Background Image.Image"=w562:dbl[][])
        n259 = Array Size(array=w562) -> (size(s)=w561:i32[])
        n260 = Equal To 0?(x=w561) -> (x = 0?=w560:bool[])
        n261 = And Array Elements(Boolean array=w560) -> (logical AND=w559:bool)
        n262 = case shown="False" w559 {
          tunnel: [w573 w586] -> w571
          tunnel: w568 -> [w578 _]
          tunnel: w564 -> [w576 w586]
          tunnel: w562 -> [w575 _]
          frame False {
            w583 = "\r\n"
            n263 = property on="Path/File" class="Path"(error in=w576) -> (error out=w572:errorcluster, "Value"=w582:path)  [unwired: 1 in, 1 out]
            n264 = Path To String(path=w582) -> (string=w581:string)
            n265 = Array To Spreadsheet String(array=w575, 3:"%9" ("format string")) -> (spreadsheet string=w579:string)  [unwired: 1 in]
            n266 = Concatenate Strings("File: " ("string"), w581, w583, "Background Image used by the ", w578, w583, w583, w579) -> (w574:string)
            n267 = call "PH_DataViewer.write Data to Harddisk.vi"("error in"=w572, "String"=w574) -> ("error out"=w573:errorcluster)
          }
          frame True {
            n268 = One Button Dialog(message="There is no image to save!") -> ()  [unwired: 1 in, 1 out]
          }
        }
      }
      event "Export Data BRM": Value Change {
        w604 = "\r\n"
        n269 = event-data() -> ()  [unwired: 1 in, 1 out]
        n270 = property on="Backreflection Measurement" class="Ring (strict)"(error in=w610) -> (error out=w609:errorcluster, "Value"=w608:u16)  [unwired: 1 in, 1 out]
        n271 = property on="Backreflection Meas" class="Arr (strict)"(error in=w609) -> (error out=w587:errorcluster, "Value"=w607:T2[])  [unwired: 1 in, 1 out]
        n272 = Index Array(array=w607, index=w608) -> (element=w611:T2)
        n273 = Unbundle By Name(w611) -> ("Instance"=w601:string, "Snapshot: Date"=w599:string, "Snapshot: Time"=w598:string, "Waveform Data"=w606:T51)
        n274 = Unbundle By Name(w606) -> ("X Increment"=w590:dbl, "Waveform Array"=w589:dbl[])
        n275 = Array Size(array=w589) -> (size(s)=w591:i32)
        n276 = for {
          N: w591 -> [_]
          tunnel: w590 -> [w615]
          tunnel: [w613] -> w595 mode=indexing
          i -> [w614]
          n277 = Multiply(x=w615, y=w614) -> (x*y=w613:dbl)
        }
        n278 = Build Array(w595, w589) -> (w594:dbl[][])
        n279 = Transpose 2D Array(2D array=w594) -> (transposed array=w593:dbl[][])
        n280 = Array To Spreadsheet String(array=w593, 3:"%f" ("format string")) -> (spreadsheet string=w588:string)  [unwired: 1 in]
        n281 = Concatenate Strings("Information saved with \"" ("string"), w601, "\" on " ("string"), w599, " at " ("string"), w598, w604, "1st column: Distance low Energy Signal [m]; 2nd column: low Energy Signal [V]; 3rdt column: Distance high Energy Signal [m]; 4th column: high Energy Signal [V]" ("string"), w604, w604, w588) -> (w605:string)
        n282 = call "PH_DataViewer.write Data to Harddisk.vi"("error in"=w587, "String"=w605) -> ("error out"=w603:errorcluster)
      }
      event "Export OO Spectro Data": Value Change {
        n283 = event-data() -> ()  [unwired: 1 in, 1 out]
        n284 = property on="OO Spectrometer Instancelist" class="Ring (strict)"(error in=w628) -> (error out=w626:errorcluster, "Value"=w627:u16)  [unwired: 1 in, 1 out]
        n285 = property on="OO Spectrometer" class="Arr (strict)"(error in=w626) -> (error out=w624:errorcluster, "Value"=w625:T52[])  [unwired: 1 in, 1 out]
        n286 = Index Array(array=w625, index=w627) -> (element=w629:T52)
        n287 = Unbundle By Name(w629) -> ("Instance"=w622:string, "Date"=w620:string, "Time"=w621:string, "Wavelength Bins"=w618:dbl[], "Spectrum by Pixels"=w617:dbl[])
        n288 = Build Array(w618, w617) -> (w619:dbl[][])
        n289 = Transpose 2D Array(2D array=w619) -> (transposed array=w616:dbl[][])
        n290 = call "PH_OceanOpticsSpectrometer.save Data to Harddisk.vi"("Instance name"=w622, "Recording Date"=w620, "Recording Time"=w621, "Data"=w616, "error in"=w624) -> ("error out"=w623:errorcluster)  [unwired: 14 in]
      }
      event "Powermeter": Value Change {
        n291 = event-data() -> ("NewVal"=w651:u16)  [unwired: 1 in]
        n292 = property on="Powermeters" class="Arr (strict)"(error in=w649) -> (error out=w631:errorcluster, "Value"=w652:T53[])  [unwired: 1 in, 1 out]
        n293 = Index Array(array=w652, index=w651) -> (element=w650:T53)
        n294 = Unbundle By Name(w650) -> ("Snapshot: Date"=w648:string, "Snapshot: Time"=w647:string, "Serial Number"=w646:string, "Current Value"=w645:dbl, "Current Value Unit"=w644:string, "Scaling Factor"=w643:dbl, "Trigger Level"=w642:dbl, "Device State"=w641:T54)
        n295 = property on="Date Powermeter" class="Str"(error in=w631, "Value"=w648) -> (error out=w640:errorcluster)  [unwired: 1 in, 1 out]
        n296 = property on="Time Powermeter" class="Str"(error in=w640, "Value"=w647) -> (error out=w639:errorcluster)  [unwired: 1 in, 1 out]
        n297 = property on="Serial Number" class="Str"(error in=w639, "Value"=w646) -> (error out=w638:errorcluster)  [unwired: 1 in, 1 out]
        n298 = property on="Current Value" class="DigNum (strict)"(error in=w638, "Value"=w645) -> (error out=w637:errorcluster)  [unwired: 1 in, 1 out]
        n299 = property on="Unit" class="Str"(error in=w637, "Value"=w644) -> (error out=w636:errorcluster)  [unwired: 1 in, 1 out]
        n300 = property on="Scaling Factor" class="DigNum (strict)"(error in=w636, "Value"=w643) -> (error out=w635:errorcluster)  [unwired: 1 in, 1 out]
        n301 = property on="Trigger Level" class="DigNum (strict)"(error in=w635, "Value"=w642) -> (error out=w634:errorcluster)  [unwired: 1 in, 1 out]
        n302 = property on="Status Powermeter" class="ColBox"(error in=w634, "Value"=w641) -> (error out=w633:errorcluster)  [unwired: 1 in, 1 out]
      }
      event "Backreflection Measurement": Value Change {
        n303 = event-data() -> ("NewVal"=w653:u16)  [unwired: 1 in, 5 out]
        n304 = property on="Backreflection Meas" class="Arr (strict)"(error in=w665) -> (error out=w662:errorcluster, "Value"=w664:T2[])  [unwired: 1 in, 1 out]
        n305 = Index Array(array=w664, index=w653) -> (element=w667:T2)
        n306 = Unbundle By Name(w667) -> ("Snapshot: Date"=w663:string, "Snapshot: Time"=w661:string, "Waveform Data.Waveform Array"=w657:dbl[], "Waveform Data.X Increment"=w656:dbl)
        n307 = call "PH_BackreflectionMeas.create waveform.vi"("dt"=w656, "Y-Data"=w657) -> ("waveform out"=w655:waveform(dbl))
        n308 = property on="Date BRM" class="Str"(error in=w662, "Value"=w663) -> (error out=w660:errorcluster)  [unwired: 1 in, 1 out]
        n309 = property on="Time BRM" class="Str"(error in=w660, "Value"=w661) -> (error out=w659:errorcluster)  [unwired: 1 in, 1 out]
        n310 = Build Array(w655) -> (w654:waveform(dbl)[])
        n311 = property on="BRM Graph" class="WFGraph (strict)"(error in=w659, "Value"=w654) -> (error out=w658:errorcluster)  [unwired: 1 in, 1 out]
      }
      event "OO Spectrometer Instancelist": Value Change {
        n312 = event-data() -> ("NewVal"=w668:u16)  [unwired: 1 in, 5 out]
        n313 = property on="OO Spectrometer" class="Arr (strict)"(error in=w679) -> (error out=w677:errorcluster, "Value"=w678:T52[])  [unwired: 1 in, 1 out]
        n314 = Index Array(array=w678, index=w668) -> (element=w681:T52)
        n315 = Unbundle By Name(w681) -> ("Date"=w673:string, "Time"=w672:string, "Wavelength Bins"=w670:dbl[], "Spectrum by Pixels"=w669:dbl[])
        n316 = property on="Date OO Spectro" class="Str"(error in=w677, "Value"=w673) -> (error out=w676:errorcluster)  [unwired: 1 in, 1 out]
        n317 = property on="Time OO Spectro" class="Str"(error in=w676, "Value"=w672) -> (error out=w675:errorcluster)  [unwired: 1 in, 1 out]
        n318 = Bundle("Wavelength Bins"=w670, "Spectrum by Pixels"=w669) -> (w671:T48)  [unwired: 1 in]
        n319 = property on="OO Spectrum" class="XYGraph (strict)"(error in=w675, "Value"=w671) -> (error out=w674:errorcluster)  [unwired: 1 in, 1 out]
      }
      event "Power Unit": Value Change {
        n320 = event-data() -> ("NewVal"=w692:u16)  [unwired: 1 in]
        n321 = property on="PP PUs" class="Arr (strict)"(error in=w696) -> (error out=w719:errorcluster, "Value"=w683:T55[])  [unwired: 1 in, 1 out]
        n322 = Index Array(array=w683, index=w692) -> (element=w691:T55)
        n323 = Unbundle By Name(w691) -> ("Gate Gen Channel"=w690:string)
        n324 = Equal?(x=w690, y="N/A") -> (x = y?=w688:bool)
        n325 = Select(t=u8 2, s=w688, f=u8 1 ("Version")) -> (s? t:f=w685:u8)
        n326 = case shown="2" w685 {
          tunnel: "PP PU Data Version 2" -> [w723 w726]
          tunnel: w683 -> [_ w725]
          tunnel: [w722 w724] -> w682
          frame 0, Default {
            n327 = Build Array(w723) -> (w722:T3[])
          }
          frame 2 {
            n328 = for {
              tunnel: w726 -> [w738]
              tunnel: w725 -> [w737] mode=indexing
              tunnel: [w727] -> w724 mode=indexing
              n329 = Unbundle By Name(w737) -> ("Instance"=w736:string, "Snapshot: Date"=w735:string, "Snapshot: Time"=w734:string, "PU in use?"=w733:bool, "Time betweeen Shots [Min]"=w732:dbl, "Waiting Time over?"=w731:bool, "Voltage [V]"=w730:dbl, "State"=w729:T56, "Timeout SM"=w728:string)
              n330 = Bundle By Name(cluster=w738, "Instance"=w736, "Snapshot: Date"=w735, "Snapshot: Time"=w734, "PU in use?"=w733, "Time betweeen Shots [Min]"=w732, "Waiting Time over?"=w731, "Voltage [V]"=w730, "State"=w729, "Timeout SM"=w728) -> (w727:T3)
            }
          }
        }
        n331 = call "PH_DataViewer.set PU GUI Elements.vi"("index"=w692, "PP PUs Vers 1"=w683, "PP PUs Vers 2"=w682, "Version"=w685) -> ("Snapshot: Date before Shot"=w721:string, "State after Shot"=w702:T4, "Snapshot: Time before Shot"=w720:string, "PU in use after Shot"=w701:bool, "PU in use before Shot"=w717:bool, "Snapshot: Time after Shot"=w700:string, "State before Shot"=w715:T4, "Waiting Time over?"=w713:bool, "Voltage [V]"=w711:dbl, "Delay [s]"=→"Delay [s]":dbl, "Gate Gen Channel"=→"Gate Gen Chan":string, "Timeout SM"=w709:string, "Time betweeen Shots [Min]"=w703:dbl, "Snapshot: Date after Shot"=w699:string)  [unwired: 7 in, 3 out]
        n332 = property on="Date PU before Shot" class="Str"(error in=w719, "Value"=w721) -> (error out=w718:errorcluster)  [unwired: 1 in, 1 out]
        n333 = property on="Time PU before Shot" class="Str"(error in=w718, "Value"=w720) -> (error out=w716:errorcluster)  [unwired: 1 in, 1 out]
        n334 = property on="in use before Shot" class="Bool (strict)"(error in=w716, "Value"=w717) -> (error out=w714:errorcluster)  [unwired: 1 in, 1 out]
        n335 = property on="State before Shot" class="Ring (strict)"(error in=w714, "Value"=w715) -> (error out=w712:errorcluster)  [unwired: 1 in, 1 out]
        n336 = property on="Waiting Time over" class="Bool (strict)"(error in=w712, "Value"=w713) -> (error out=w710:errorcluster)  [unwired: 1 in, 1 out]
        n337 = property on="Voltage [V]" class="DigNum (strict)"(error in=w710, "Value"=w711) -> (error out=w695:errorcluster)  [unwired: 1 in, 1 out]
        n338 = property on="Timeout SM" class="Str"(error in=w695, "Value"=w709) -> (error out=w708:errorcluster)  [unwired: 1 in, 1 out]
        n339 = property on="Waiting Time [Min]" class="DigNum (strict)"(error in=w708, "Value"=w703) -> (error out=w707:errorcluster)  [unwired: 1 in, 1 out]
        n340 = property on="State after Shot" class="Ring (strict)"(error in=w707, "Value"=w702) -> (error out=w706:errorcluster)  [unwired: 1 in, 1 out]
        n341 = property on="in use after Shot" class="Bool (strict)"(error in=w706, "Value"=w701) -> (error out=w705:errorcluster)  [unwired: 1 in, 1 out]
        n342 = property on="Time PU after Shot" class="Str"(error in=w705, "Value"=w700) -> (error out=w704:errorcluster)  [unwired: 1 in, 1 out]
        n343 = property on="Date PU after Shot" class="Str"(error in=w704, "Value"=w699) -> (error out=w698:errorcluster)  [unwired: 1 in, 1 out]
      }
      event "Cameras": Value Change {
        n344 = event-data() -> ("NewVal"=w758:u16)  [unwired: 1 in]
        n345 = property on="Cams" class="Arr (strict)"(error in=w754) -> (error out=w756:errorcluster, "Value"=w759:T49[])  [unwired: 1 in, 1 out]
        n346 = call "PH_DataViewer.get i attribute.vi"("i ref in"=w755, "error in (no error)"=w756) -> ("i ref out"=w739:refnum<vi>, "i attribute"=w761:T32, "error out"=w746:errorcluster)  [unwired: 15 in]
        n347 = Index Array(array=w759, index=w758) -> (element=w757:T49)
        n348 = Unbundle By Name(w761) -> ("Images.CAM"=w760:cluster{string, u32})
        n349 = Unbundle By Name(w757) -> ("Img taken: Date"=w753:string, "Img Taken: Time"=w752:string, "Cam Settings"=w751:T50, "Image"=w749:sgl[][], "Cam.Trigger"=w750:T19)
        n350 = call <vilib>:"IMAQ Image Cluster to Image Datatype.vi"("Image"=w760) -> ("Image (dup)"=w747:T21)
        n351 = call "IMAQ ArrayToImage"("Image Pixels (Float)"=w749, "error in (no error)"=w746, "Image"=w747) -> ("error out"=w745:errorcluster, "Image Out"=w748:T21)  [unwired: 7 in]
        n352 = property on="Cam Image" class="ImageControl"(error in=w745, "Value"=w748) -> (error out=w744:errorcluster)  [unwired: 1 in, 1 out]
        n353 = property on="Date Cams" class="Str"(error in=w744, "Value"=w753) -> (error out=w743:errorcluster)  [unwired: 1 in, 1 out]
        n354 = property on="Time Cams" class="Str"(error in=w743, "Value"=w752) -> (error out=w742:errorcluster)  [unwired: 1 in, 1 out]
        n355 = property on="Cam Settings" class="Clust (strict)"(error in=w742, "Value"=w751) -> (error out=w741:errorcluster)  [unwired: 1 in, 1 out]
        n356 = property on="Cam Trigger" class="Clust (strict)"(error in=w741, "Value"=w750) -> (error out=w740:errorcluster)  [unwired: 1 in, 1 out]
      }
      event "Operators": Value Change {
        n357 = event-data() -> ("NewVal"=w770:u16)  [unwired: 1 in]
        n358 = property on="Img Operators" class="Arr (strict)"(error in=w771) -> (error out=w768:errorcluster, "Value"=w772:T5[])  [unwired: 1 in, 1 out]
        n359 = Index Array(array=w772, index=w770) -> (element=w764:T5)
        n360 = call "PH_DataViewer.set Img Op GUI elements.vi"("i ref in"=w769, "Img Operator Data"=w764, "error in (no error)"=w768) -> ("i ref out"=w767:refnum<vi>, "error out"=w763:errorcluster)  [unwired: 15 in]
        n361 = Unbundle By Name(w764) -> ("Trace Analysis.on"=w765:bool, "Trace Analysis.Traces"=w766:T46)
        n362 = case shown="False" w765 {
          tunnel: w766 -> [_ w794]
          tunnel: w763 -> [w775 w791]
          tunnel: [w773 w789] -> w762
          frame False {
            w776 = cluster{"Index":sgl[], dbl[]}[] [] ("Major Trace")
            n363 = property on="Major Trace" class="XYGraph (strict)"(error in=w775, "Value"=w776) -> (error out=w774:errorcluster)  [unwired: 1 in, 1 out]
            n364 = property on="Major Trace" class="XYGraph (strict)"(error in=w774, "Value"=w776) -> (error out=w773:errorcluster)  [unwired: 1 in, 1 out]
          }
          frame True {
            n365 = Index Array(array=w794) -> (element #1=w793:T47, element #2=w792:T47)  [unwired: 2 in]
            n366 = Unbundle By Name(w793) -> ("XScaleName"=w788:string, "Y Scale Minimum"=w787:sgl, "Y Scale Maximum"=w786:sgl, "X Scale Minimum"=w785:sgl, "X Scale Maximum"=w784:sgl, "Traces"=w783:cluster{"Index":sgl[], "Trace":dbl[]}[])
            n367 = property on="Minor Trace" class="XYGraph (strict)"(error in=w791, "X Scale.Name Label.Text"=w788, "Y Scale.Range:Minimum"=w787, "Y Scale.Range:Maximum"=w786, "X Scale.Range:Minimum"=w785, "X Scale.Range:Maximum"=w784, "Value"=w783) -> (error out=w790:errorcluster)  [unwired: 1 in, 1 out]
            n368 = Unbundle By Name(w792) -> ("XScaleName"=w782:string, "Y Scale Minimum"=w781:sgl, "Y Scale Maximum"=w780:sgl, "X Scale Minimum"=w779:sgl, "X Scale Maximum"=w778:sgl, "Traces"=w777:cluster{"Index":sgl[], "Trace":dbl[]}[])
            n369 = property on="Minor Trace" class="XYGraph (strict)"(error in=w790, "X Scale.Name Label.Text"=w782, "Y Scale.Range:Minimum"=w781, "Y Scale.Range:Maximum"=w780, "X Scale.Range:Minimum"=w779, "X Scale.Range:Maximum"=w778, "Value"=w777) -> (error out=w789:errorcluster)  [unwired: 1 in, 1 out]
          }
        }
      }
    }
    "loop counter" <- w54
  }
  "error out" <- w2
  n370 = call "PH_Interaction.Super Destroy Me.vi"("i ref out"=w3) -> ()
